vi "SIM control.vi"(11 "User":string="unknown-LAGSIM-user") -> ()   [LabVIEW 2018]
uses:
  <vilib>/DAQmx/write.llb/DAQmx Write (Digital Bool 1Line 1Point).vi
  <vilib>/DAQmx/create/channels.llb/DAQmx Create Channel (DO-Digital Output).vi
  <vilib>/DAQmx/write.llb/DAQmx Write (Analog DBL 1Chan 1Samp).vi
  <vilib>/DAQmx/write.llb/DAQmx Write (Digital 1D Bool 1Chan 1Samp).vi
  <vilib>/DAQmx/read.llb/DAQmx Read (Digital Bool 1Line 1Point).vi
  <vilib>/DAQmx/create/channels.llb/DAQmx Create Channel (AO-Voltage-Basic).vi
  <vilib>/DAQmx/read.llb/DAQmx Read (Analog DBL 1Chan 1Samp).vi
  <vilib>/Utility/file.llb/Write To Spreadsheet File (string).vi
  <vilib>/Utility/file.llb/Read From Spreadsheet File (string).vi
  <vilib>/Platform/browser.llb/Open URL in Default Browser (string).vi
  <vilib>/DAQmx/create/channels.llb/DAQmx Create Channel (AI-Voltage-Basic).vi
  <vilib>/Instr/_visa.llb/VISA Configure Serial Port (Instr).vi
  <vilib>/DAQmx/create/channels.llb/DAQmx Create Channel (DI-Digital Input).vi
panel:
  out "Laser Cluster":T1
  in  "y-move":bool
  in  "x-move":bool
  in  "y-rel (um)":dbl
  in  "x-rel (um)":dbl
  in  "Labstep API_Key":string="ZDNlNzY2YTYwNjk2YjY0Y2E4OGZhMGNiMDYxMWJkZjVjNWMwMjMzOQ=="
  in  "Live OS Channel Cluster":T2
  in  "Optosplit":bool
  in  "SIM Frames":i16=9
  in  "Bleach-\nsave ratio":dbl=1.0 min=0.0 max=1.0 step=0.1 format="%.2f"
  out "Current filter":string
  out "Current bookmark":i32
  out "TIRF Mode N":T3
  in  "Preview view":T4(radio)
  in  "Exposure\n(ms)":u32=100 min=1 max=2000 step=5
  in  "Channel":T5(radio)
  in  "Live on":bool
  out "Exposure times N":dbl[](array[numeric])
  out "Current piezo position (V)":dbl min=0.0 max=10.0 step=0.01 format="%_4g"
  out "ASI VISA resource name":refnum<visa-resource-name>="COM17"
  out "Voltage TIMEOUT (V)":dbl
  in  "stop":bool
  in  "Tab Control":T6(tab)=enum."-- Acquire --"
  in  "Clear table":bool
  in  "Create grid":bool
  in  "Load bkmk table":bool
  in  "Save bkmk table":bool
  in  "Delete bkmk":bool
  in  "Add bkmk":bool
  in  "Bookmark List":i32(listbox)=-1
  out "Output Voltage":dbl
  out "Total Sweep Images:":i16=360
  in  "Sweep Pattern":u8(ring)=21 items=["P9 0deg"=21, "P9 60deg"=22, "P9 120deg"=23, "P12 0deg"=24, "P12 60deg"=25, "P12 120deg"=26, "P15 0deg"=27, "P15 60deg"=28, "P15 120deg"=29]
  in  "Max V":dbl=1.0 min=-1.0 max=1.0
  in  "Min V":dbl=-1.0 min=-1.0 max=1.0
  in  "Sweep":bool caption="LCVR sweep"
  in  "V. steps":i16=40
  out "Step index:":i16
  in  "Voltages:":dbl[][](array[numeric])=[[0.09, 0.13, 0.16], [0.44, 0.52, 0.62], [-0.25, -0.28, -0.3]]
  in  "Filter Optosplit":i8=7 min=1 max=10 step=1
  in  "Filter 561":i8=3 min=1 max=10 step=1
  in  "Filter 640":i8=2 min=1 max=10 step=1
  in  "Filter 488":i8=4 min=1 max=10 step=1
  in  "Manual SLM mode":bool
  in  "RO":u8=7 max=41 step=1
  out "SLM status":i16
  out "RO #":u8=49
  out "SLM State":string="Active"
  in  "Z-move method":u16(ring)=1 items=["Analogue", "Serial"]
  out "Current RO":u8=7
  in  "use z offset":bool
  out "Current z-position (um)":dbl min=0.0 max=10.0 step=0.01 format="%_4g"
  in  "Z offset (um)":dbl[](array[numeric])=[0.0, -0.3, 84.0] min=0.0 max=360.0 step=0.1 format="%0.3f"
  out "Current z #":i16=1
  in  "z0 (um)":dbl step=0.01 format="%.2f"
  in  "Post to logbook":bool
  in  "Logbook entry":string
  in  "Open Logbook":bool
  in  "LED intensity":dbl min=0.0 max=100.0 step=1.0
  in  "ASI Unlock":bool
  in  "ASI Set Lock":bool
  in  "TIRF Info button":bool
  in  "640-OS":bool
  in  "561-OS":bool
  in  "488-OS":bool
  in  "Exp OS":string="100"
  in  "Ch3 TIRF":bool
  in  "Ch2 TIRF":bool
  in  "Ch1 TIRF":bool
  in  "Widefield?":bool
  in  "#bookmarks":i16 min=0 step=1
  in  "Acquire":bool
  in  "#Channels":i16=1 min=1 max=3 step=1
  in  "#t-frames":i16=1 min=1 step=1
  out "Total\nFrames":i16=36
  out "Current \nFrame":i32
  in  "Ch 1":T5(radio)
  in  "Ch 2":T5(radio)=enum."Radio Selection 2"
  in  "Ch 3":T5(radio)=enum."Radio Selection 3"
  in  "t-interval":u32 max=1000 step=1
  in  "Int unit":enum16{"ms", "s", "min"}(ring)
  in  "Exp 0":u32=100 caption="Exposure (ms) 2" min=1 max=2000 step=5
  in  "Exp 1":u32=100 caption="Exposure (ms) 2" min=1 max=2000 step=5
  in  "Exp 2":u32=100 caption="Exposure (ms) 2" min=1 max=2000 step=5
  in  "#z-planes":i16=1 min=1 step=1
  in  "z-step (um)":dbl=1.0
  out "Z move":bool
  out "Ch N":T7={"Ch 0"=enum."Radio Selection 1", "Ch 1"=enum."Radio Selection 2", "Ch 2"=enum."Radio Selection 3"}
  # "LIVE!"
  # "ADVANCED"
  # "Channel Variable Holders"
  # "Pockels Voltage Sweep"
  # "Pockels Voltage Settings"
  # "488           561            640"
  # "Rot 1\n\nRot 2\n\nRot 3"
  # "Filter position"
  # "ASI stage comms"
  # "488"
  # "640"
  # "Opto"
  # "561"
  # "Manual SLM control"
  # "Piezo offset"
  # "Channel #"
  # "Use this space to report any bugs, problems, or anything\nelse you like to the logbook."
  # "ASI Autofocus"
  # "UNDER DEVELOPMENT!!!"
  # "O/S"
  # "TIRF:"
  # "TIRF:"
  # "TIRF:"
  # "Wave-\nlength:"
  # "Exposure\ntime (ms):"
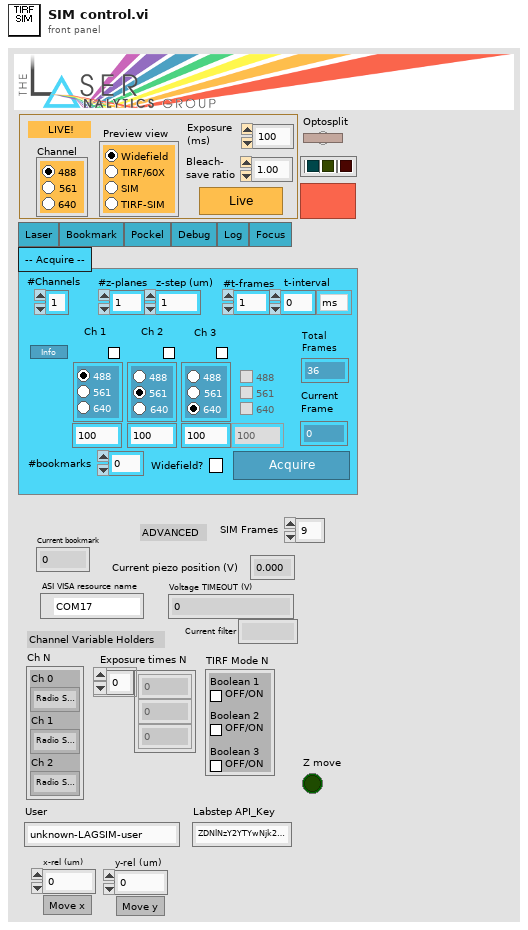
[diagram p1: front panel]
types:
  T1 = cluster{"488 indicator":bool, "488 indicator 3":bool, "488 indicator 2":bool}
  T2 = cluster{"488 OS live":bool, "640 OS live":bool, "561 OS live":bool}
  T3 = cluster{"Boolean 1":bool, "Boolean 2":bool, "Boolean 3":bool}
  T4 = enum32{"Radio Selection 1", "Radio Selection 2", "Radio Selection 3", "Radio Selection 4"}
  T5 = enum32{"Radio Selection 1", "Radio Selection 2", "Radio Selection 3"}
  T6 = enum32{"Laser", "Bookmark", "Pockel", "Debug", "Log", "Focus", "-- Acquire --"}
  T7 = cluster{"Ch 0":enum32{"Radio Selection 1", "Radio Selection 2", "Radio Selection 3"}, "Ch 1":enum32{"Radio Selection 1", "Radio Selection 2", "Radio Selection 3"}, "Ch 2":enum32{"Radio Selection 1", "Radio Selection 2", "Radio Selection 3"}}
  T8 = cluster{"Ch 1":enum32{"Radio Selection 1", "Radio Selection 2", "Radio Selection 3"}, "Ch 2":enum32{"Radio Selection 1", "Radio Selection 2", "Radio Selection 3"}, "Ch 3":enum32{"Radio Selection 1", "Radio Selection 2", "Radio Selection 3"}}
  T9 = cluster{"Ch1 TIRF":bool, "Ch2 TIRF":bool, "Ch3 TIRF":bool}
  T10 = cluster{"User":string, "Total\nFrames":i16, "#Channels":i16, "#t-frames":i16, "#z-planes":i16, "#bookmarks":i16, "Ch N":cluster{"Ch 0":enum32{"Radio Selection 1", "Radio Selection 2", "Radio Selection 3"}, "Ch 1":enum32{"Radio Selection 1", "Radio Selection 2", "Radio Selection 3"}, "Ch 2":enum32{"Radio Selection 1", "Radio Selection 2", "Radio Selection 3"}}, "Exposure times N":dbl[], "TIRF Mode N":cluster{"Boolean 1":bool, "Boolean 2":bool, "Boolean 3":bool}, "Optosplit":bool, "Widefield?":bool, "t-interval":u32, "RingText.Text":string, "z-step (um)":dbl, i32}
  T11 = enum8{"Enabled", "Disabled", "Disabled and Grayed Out"}
  T12 = cluster{"data[0]":bool, "data[1]":bool, "data[2]":bool}
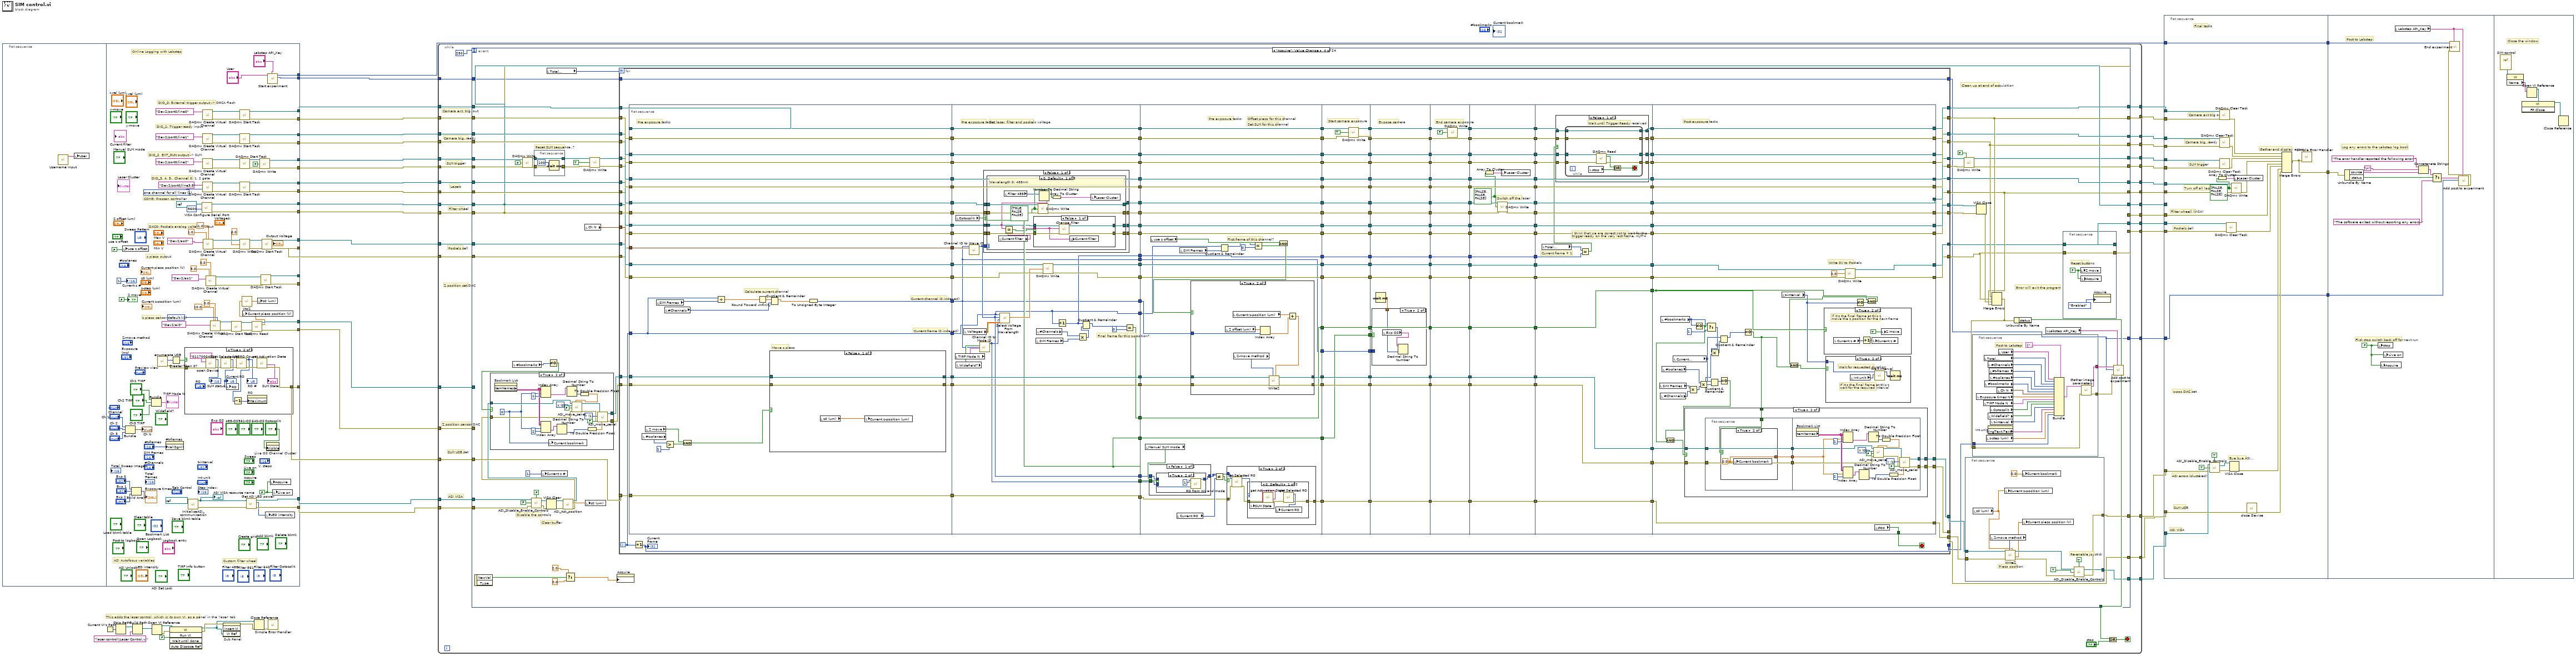
[diagram p0: block diagram]
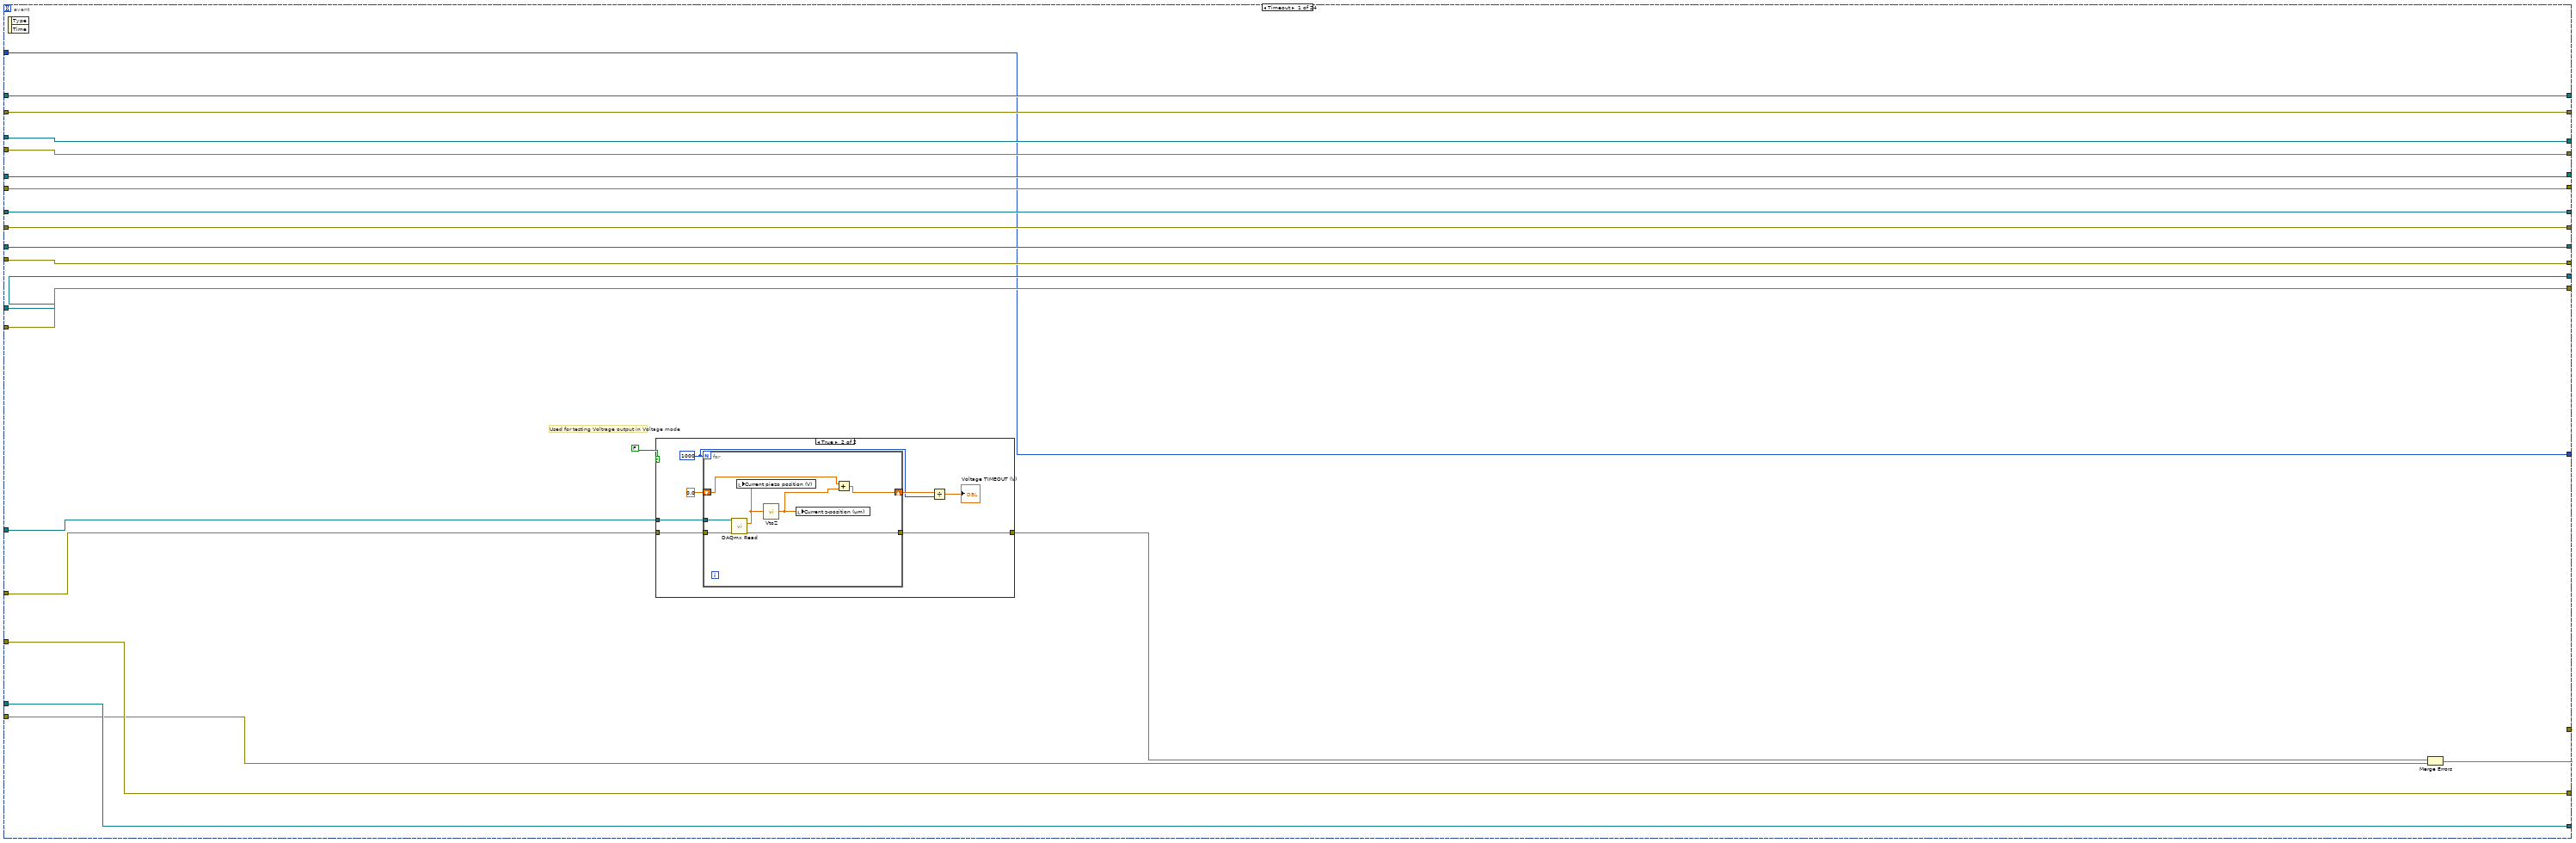
[diagram p2: hidden frame]
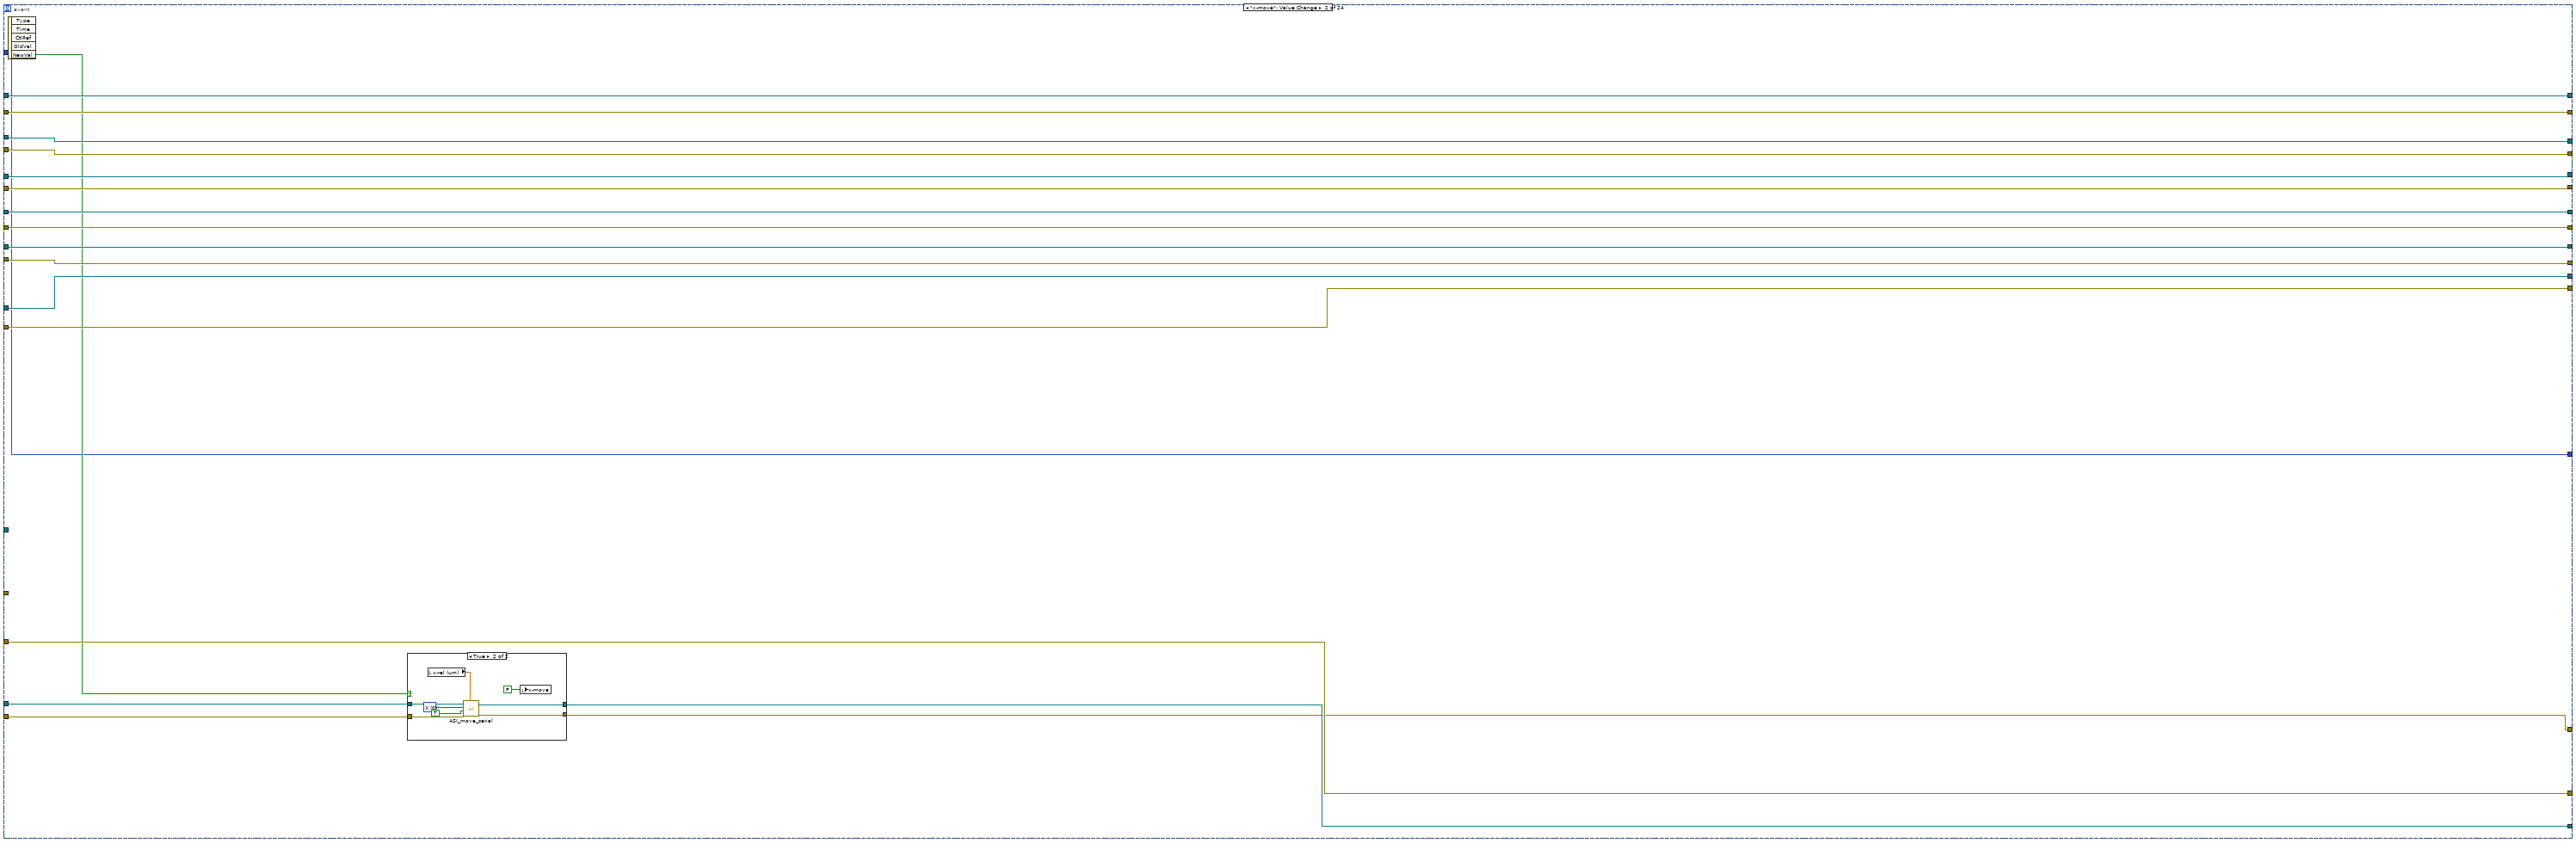
[diagram p4: hidden frame]
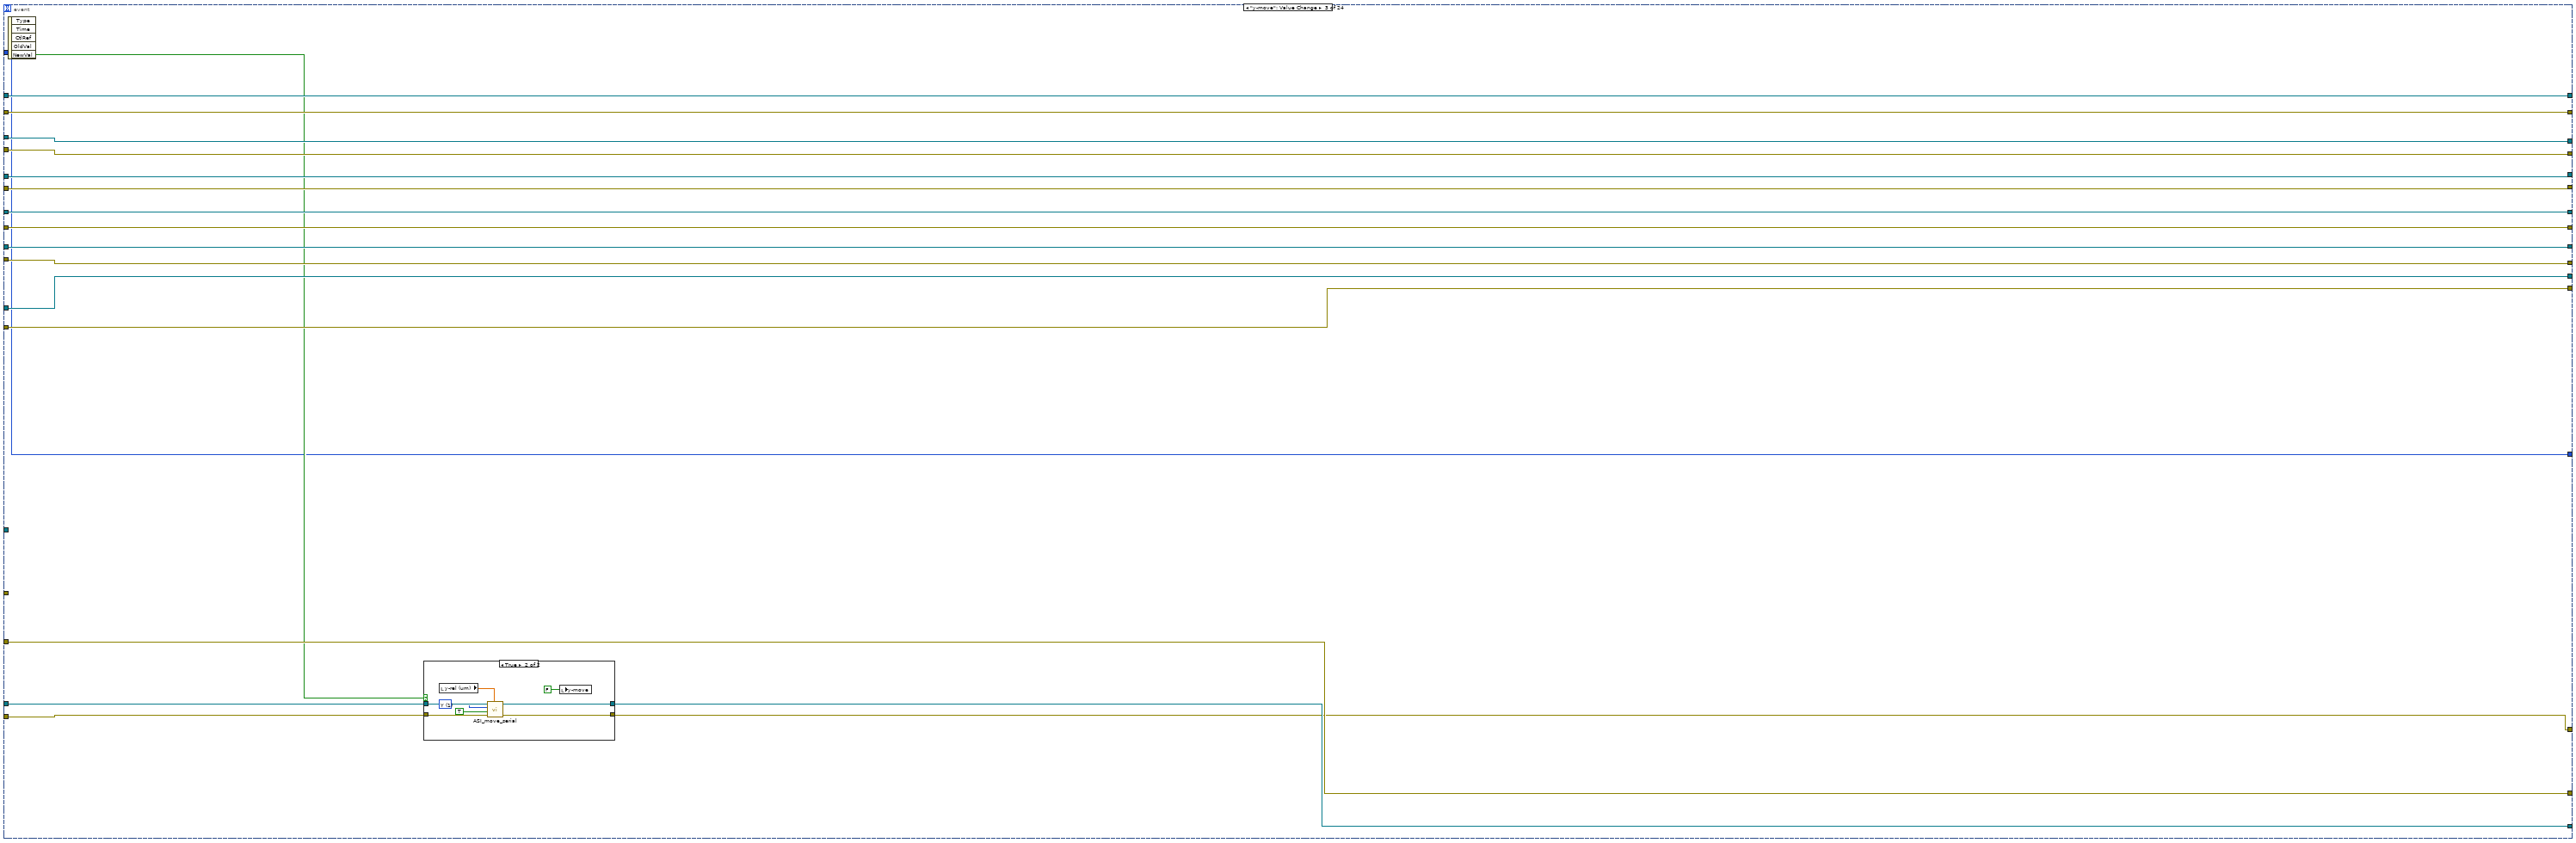
[diagram p6: hidden frame]
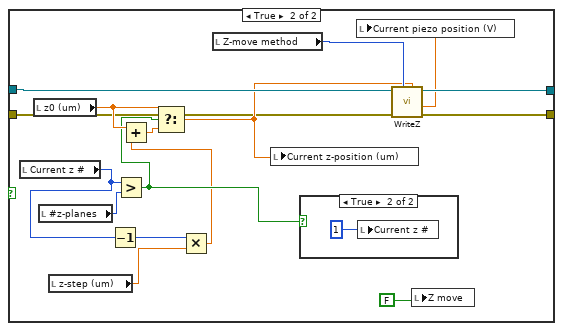
[diagram p9: hidden frame]
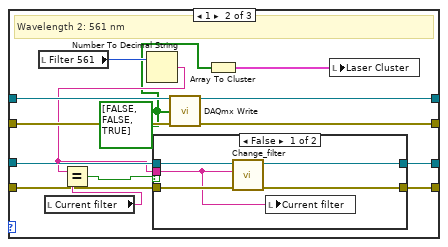
[diagram p12: hidden frame]
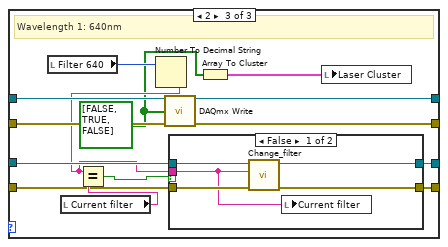
[diagram p14: hidden frame]
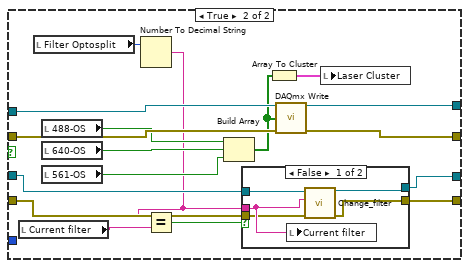
[diagram p16: hidden frame]
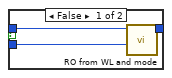
[diagram p20: hidden frame]
diagram:
  # "This adds the laser control, which is its own VI, as a panel in the 'laser' tab"
  n1 = flat-sequence {
    tunnel: [w136] -> w34
    tunnel: [w135] -> w48
    tunnel: [w131] -> w33
    tunnel: [w130] -> w46
    tunnel: [w121] -> w43
    tunnel: [w120] -> w42
    tunnel: [w111] -> w30
    tunnel: [w110] -> w39
    tunnel: [w109] -> w32
    tunnel: [w108] -> w36
    tunnel: [w99] -> w31
    tunnel: [w98] -> w35
    tunnel: [w81] -> w29
    tunnel: [w82] -> w28
    tunnel: [w88] -> _
    tunnel: [w87] -> _
    tunnel: [w75] -> w25
    tunnel: [w58] -> w24
    tunnel: [w56] -> w19
    tunnel: [w52] -> w1
    tunnel: [w51] -> w4
    frame #0 {
      n2 = call "Username Input.vi"() -> ("Username output"=w50:string)  [unwired: 11 in]
      n3 = local write "User"(w50) -> ()
    }
    frame #1 {
      w74 = FALSE ("Live mode")
      w91 = -1 items=["default"=-1, "RSE"=10083, "NRSE"=10078, "Differential"=10106, "Pseudodifferential"=12529] ("input terminal configuration")
      w106 = 1 items=["one channel for each line", "one channel for all lines"] ("line grouping")
      # "Custom filter wheel"
      # "ASI Autofocus variables"
      # "Online Logging with Labstep"
      # "z piezo sensor"
      # "z piezo output"
      # "COM5: Proscan controller"
      # "DIO_3, 4, 5:  Channel 0, 1, 2 gate"
      # "DIO_2  EXT_RUN output -> SLM"
      # "DAC0: Pockels analog voltage output"
      # "DIO_1: Trigger ready input"
      # "DIO_0: External trigger output -> ORCA Flash"
      n4 = local write "use z offset"(FALSE ("use z offset")) -> ()
      n5 = Bundle("Ch 1"="Ch 1", "Ch 2"="Ch 2", "Ch 3"="Ch 3") -> (→"Ch N":T8)  [unwired: 1 in]
      n6 = Build Array("Exp 0", "Exp 1", "Exp 2") -> (→"Exposure times N":u32[])
      n7 = Bundle("Ch1 TIRF"="Ch1 TIRF", "Ch2 TIRF"="Ch2 TIRF", "Ch3 TIRF"="Ch3 TIRF") -> (→"TIRF Mode N":T9)  [unwired: 1 in]
      n8 = call <userlib>:"enumerate USB.vi"() -> ("error out"=w76:errorcluster, "function return"=w78:i16)  [unwired: 9 in, 1 out]
      n9 = property on="#t-frames" class="DigNum (strict)"("Val(Sgnl)"="#t-frames") -> ()  [unwired: 2 in, 2 out]
      n10 = Greater Than 0?(x=w78) -> (x > 0?=w77:bool)
      n11 = case shown="True" w77 {
        tunnel: w76 -> [w141 w152]
        tunnel: [w140 w147] -> w75
        frame False {
          n12 = call <userlib>:"close Device.vi"("error in (no error)"=w141) -> ("error out"=w140:errorcluster)  [unwired: 9 in, 1 out]
        }
        frame True {
          n13 = call <userlib>:"open Device.vi"("error in (no error)"=w152, "identifier"="0117000451") -> ("error out"=w149:errorcluster, "function return"=→"SLM status":i16)  [unwired: 8 in]
          n14 = call <userlib>:"get Selected RO.vi"("error in (no error)"=w149) -> ("error out"=w148:errorcluster, "selectedRO"=w144:u8)  [unwired: 8 in, 1 out]
          "Current RO" <- w144
          n15 = local write "RO"(w144) -> ()
          n16 = call <userlib>:"get RO Count.vi"("error in (no error)"=w148) -> ("error out"=w146:errorcluster, "count"=w143:u8)  [unwired: 8 in, 1 out]
          "RO #" <- w143
          n17 = Decrement(x=w143) -> (x-1=w142:u8)
          n18 = property on="RO" class="DigNum (strict)"("Maximum"=w142) -> ()  [unwired: 2 in, 2 out]
          n19 = call <userlib>:"get Activation State.vi"("error in (no error)"=w146) -> ("error out"=w147:errorcluster, "String"=→"SLM State":string)  [unwired: 7 in, 2 out]
        }
      }
      n20 = call "InitialiseASI_communication.vi"("COM port"=refnum<visa-resource-name> "COM17") -> ("error out"=w57:errorcluster, "VISA resource name out"=w59:refnum<visa-resource-name>)  [unwired: 3 in]
      "ASI VISA resource name" <- w59
      n21 = call-poly "VISA Configure Serial Port"("VISA resource name"=refnum<visa-resource-name> "COM5", "baud rate (9600)"=u32 9600) -> ("VISA resource name out"=w99:refnum<visa-resource-name>, "error out"=w98:errorcluster)  [unwired: 12 in]
      n22 = call-poly <vilib>:"DAQmx Create Virtual Channel.vi"("lines"=tag "Dev2/port0/line0") -> ("task out"=w138:refnum<k21>, "error out"=w139:errorcluster)  [unwired: 13 in]
      n23 = call-poly <vilib>:"DAQmx Create Virtual Channel.vi"("lines"=tag "Dev2/port0/line1") -> ("task out"=w133:refnum<k21>, "error out"=w132:errorcluster)  [unwired: 13 in]
      n24 = call-poly <vilib>:"DAQmx Create Virtual Channel.vi"("lines"=tag "Dev2/port0/line2") -> ("task out"=w118:refnum<k21>, "error out"=w117:errorcluster)  [unwired: 13 in]
      n25 = call-poly <vilib>:"DAQmx Create Virtual Channel.vi"("lines"="Dev2/port0/line3:5", "line grouping"=w106) -> ("task out"=w116:refnum<k21>, "error out"=w115:errorcluster)  [unwired: 12 in]
      n26 = call-poly <vilib>:"DAQmx Create Virtual Channel.vi"("maximum value"=1.0, "minimum value"=-1.0, "physical channels"=tag "Dev2/ao0") -> ("task out"=w124:refnum<k21>, "error out"=w123:errorcluster)  [unwired: 11 in]
      n27 = call-poly <vilib>:"DAQmx Create Virtual Channel.vi"("maximum value"=5.0, "minimum value"=0.0, "physical channels"=tag "Dev2/ao1") -> ("task out"=w94:refnum<k21>, "error out"=w93:errorcluster)  [unwired: 11 in]
      n28 = call-poly <vilib>:"DAQmx Create Virtual Channel.vi"("maximum value"=10.0, "minimum value"=0.0, "input terminal configuration"=w91, "physical channels"=tag "Dev2/ai0" ("Physical Channel")) -> ("task out"=w86:refnum<k21>, "error out"=w85:errorcluster)  [unwired: 10 in]
      n29 = call <vilib>:"DAQmx Start Task.vi"("task/channels in"=w86, "error in"=w85) -> ("task out"=w84:refnum<k21>, "error out"=w83:errorcluster)  [unwired: 12 in]
      n30 = call <vilib>:"DAQmx Start Task.vi"("task/channels in"=w138, "error in"=w139) -> ("task out"=w136:refnum<k21>, "error out"=w135:errorcluster)  [unwired: 12 in]
      n31 = call <vilib>:"DAQmx Start Task.vi"("task/channels in"=w133, "error in"=w132) -> ("task out"=w131:refnum<k21>, "error out"=w130:errorcluster)  [unwired: 12 in]
      n32 = call <vilib>:"DAQmx Start Task.vi"("task/channels in"=w118, "error in"=w117) -> ("task out"=w114:refnum<k21>, "error out"=w113:errorcluster)  [unwired: 12 in]
      n33 = call <vilib>:"DAQmx Start Task.vi"("task/channels in"=w116, "error in"=w115) -> ("task out"=w109:refnum<k21>, "error out"=w108:errorcluster)  [unwired: 12 in]
      n34 = call-poly <vilib>:"DAQmx Write.vi"("task/channels in"=w124, "data"=0.0, "error in"=w123) -> ("task out"=w128:refnum<k21>, "error out"=w127:errorcluster)  [unwired: 10 in, 1 out]
      n35 = call "Get ASI LED power.vi"("error in"=w57, "VISA resource in"=w59) -> ("error out"=w56:errorcluster, "LED power"=w55:i32, "VISA resource name out"=w58:refnum<visa-resource-name>)  [unwired: 7 in]
      n36 = call-poly <vilib>:"DAQmx Read.vi"("task/channels in"=w84, "error in"=w83) -> ("task out"=w81:refnum<k21>, "data"=w79:dbl, "error out"=w82:errorcluster)  [unwired: 11 in]
      n37 = call "VtoZ.vi"("Voltage IN"=w79) -> ("Zpos OUT (um)"=w72:dbl)
      n38 = local write "Current piezo position (V)"(w79) -> ()
      n39 = local write "z0 (um)"(w72) -> ()
      n40 = call-poly <vilib>:"DAQmx Write.vi"("task/channels in"=w114, "data"=FALSE, "error in"=w113) -> ("task out"=w111:refnum<k21>, "error out"=w110:errorcluster)  [unwired: 10 in, 1 out]
      n41 = call <vilib>:"DAQmx Start Task.vi"("task/channels in"=w94, "error in"=w93) -> ("task out"=w88:refnum<k21>, "error out"=w87:errorcluster)  [unwired: 12 in]
      n42 = call <vilib>:"DAQmx Start Task.vi"("task/channels in"=w128, "error in"=w127) -> ("task out"=w121:refnum<k21>, "error out"=w120:errorcluster)  [unwired: 12 in]
      n43 = local write "LED intensity"(w55) -> ()
      n44 = property on="Live OS Channel Cluster" class="Clust (strict)"("Visible"="Optosplit") -> ()  [unwired: 2 in, 2 out]
      n45 = call "Start experiment.vi"("API Key"="Labstep API_Key", "Name of LAG SIM user"="User") -> ("Thread ID"=w51:i32, "Experiment ID"=w52:i32)  [unwired: 7 in, 1 out]
      n46 = local write "Acquire"(w74) -> ()
      n47 = local write "Live on"(w74) -> ()
      "Current z #" <- i16 1 ("Current z #")
      "Z move" <- FALSE ("Z move")
    }
  }
  n48 = Current VI's Path() -> (path=w14:path)
  n49 = Strip Path(path=w14) -> (stripped path=w12:path)  [unwired: 1 out]
  n50 = Build Path(base path=w12, name or relative path="laser control\\Laser Control.vi") -> (appended path=w13:path)
  n51 = Open VI Reference(vi path=w13) -> (vi reference=w17:refnum<vi>, error out=w16:errorcluster)  [unwired: 5 in]
  n52 = invoke class="VI" method="Run VI"(reference=w17, error in=w16, "Wait until done"=FALSE) -> (reference out=w7:refnum<vi>, error out=w9:errorcluster)  [unwired: 2 in, 3 out]
  n53 = invoke on="Sub Panel" class="SubPanel" method="Insert VI"(error in=w9, "VI Ref"=w7) -> (error out=w8:errorcluster)  [unwired: 2 in, 3 out]
  n54 = Close Reference(reference=w7, error in (no error)=w8) -> (error out=w11:errorcluster)
  n55 = call <vilib>:"Simple Error Handler.vi"("error in (no error)"=w11) -> ()  [unwired: 4 in, 5 out]
  n56 = while {
    tunnel: w34 -> [w190]
    tunnel: [w189] -> w49
    tunnel: w48 -> [w188]
    tunnel: [w187] -> w47
    tunnel: w33 -> [w186]
    tunnel: w46 -> [w185]
    tunnel: [w184] -> w45
    tunnel: [w168] -> w44
    tunnel: w43 -> [w183]
    tunnel: w42 -> [w182]
    tunnel: [w181] -> w41
    tunnel: [w180] -> w40
    tunnel: w30 -> [w179]
    tunnel: w39 -> [w178]
    tunnel: [w177] -> w37
    tunnel: [w176] -> w38
    tunnel: w32 -> [w175]
    tunnel: w36 -> [w174]
    tunnel: w31 -> [w173]
    tunnel: w35 -> [w172]
    tunnel: w29 -> [w171]
    tunnel: w28 -> [w170]
    tunnel: [w169] -> w27
    tunnel: [w166] -> w26
    tunnel: w25 -> [w167]
    tunnel: w24 -> [w164]
    tunnel: [w163] -> w23
    tunnel: [w162] -> w22
    tunnel: [w158] -> w21
    tunnel: [w157] -> w20
    tunnel: w19 -> [w156]
    tunnel: [w155] -> w18
    tunnel: w4 -> [w154]
    tunnel: [w153] -> w3
    stop <- w161 stop-if-true
    # "Camera trig. ready"
    # "Camera ext. trig. out"
    # "SLM trigger"
    # "Lasers"
    # "SLM USB set"
    # "Filter wheel"
    # "Pockels cell"
    # "ASI VISA"
    # "Z position sensor DAC"
    # "Z position set DAC"
    n57 = event shown="[3] \"Acquire\": Value Change" {
      selector: _ -> [_ _ _ _ _ _ _ _ _ _ _ _ _ _ _ _ _ _ _ _ _ _ _ _]
      dyn-events: _ -> [_ _ _ _ _ _ _ _ _ _ _ _ _ _ _ _ _ _ _ _ _ _ _ _]
      timeout: 250 -> [_ _ _ _ _ _ _ _ _ _ _ _ _ _ _ _ _ _ _ _ _ _ _ _]
      tunnel: w190 -> [w195 w245 w274 w358 w1092 w1130 w1528 w1578 w2099 w2102 w2128 w2162 w2190 w2230 w2285 w2305 w2322 w2352 w2370 w2394 w2423 w2449 w2474 w2492]
      tunnel: [w195 w245 w274 w356 w1092 w1114 w1528 w1574 w2099 w2102 w2128 w2162 w2190 w2230 w2285 w2305 w2322 w2352 w2370 w2394 w2423 w2449 w2474 w2492] -> w189
      tunnel: w188 -> [w196 w244 w273 w357 w1091 w1129 w1529 w1577 w2098 w2103 w2129 w2163 w2191 w2229 w2284 w2304 w2321 w2351 w2369 w2393 w2422 w2448 w2473 w2491]
      tunnel: [w196 w244 w273 w353 w1091 w1101 w1529 w1573 w2098 w2103 w2129 w2163 w2191 w2229 w2284 w2304 w2321 w2351 w2369 w2393 w2422 w2448 w2473 w2491] -> w187
      tunnel: w186 -> [w197 w242 w271 w355 w1089 w1128 w1530 w1576 w2096 w2104 w2130 w2164 w2192 w2227 w2282 w2302 w2319 w2349 w2367 w2391 w2420 w2446 w2471 w2489]
      tunnel: w185 -> [w198 w243 w272 w354 w1090 w1127 w1531 w1575 w2097 w2105 w2131 w2165 w2193 w2228 w2283 w2303 w2320 w2350 w2368 w2392 w2421 w2447 w2472 w2490]
      tunnel: [w198 w243 w272 w352 w1090 w1096 w1531 w1571 w2097 w2105 w2131 w2165 w2193 w2228 w2283 w2303 w2320 w2350 w2368 w2392 w2421 w2447 w2472 w2490] -> w184
      tunnel: [w197 w242 w271 w351 w1089 w1098 w1530 w1572 w2096 w2104 w2130 w2164 w2192 w2227 w2282 w2302 w2319 w2349 w2367 w2391 w2420 w2446 w2471 w2489] -> w168
      tunnel: w183 -> [w203 w241 w270 w349 w1088 w1136 w1538 w1559 w2095 w2112 w2138 w2172 w2200 w2226 w2281 w2301 w2318 w2348 w2366 w2390 w2419 w2445 w2470 w2488]
      tunnel: w182 -> [w204 w240 w269 w348 w1087 w1135 w1539 w1557 w2094 w2113 w2139 w2173 w2201 w2225 w2280 w2300 w2317 w2347 w2365 w2389 w2418 w2444 w2469 w2487]
      tunnel: [w203 w241 w270 w314 w1088 w1121 w1538 w1558 w2095 w2112 w2138 w2172 w2200 w2226 w2281 w2301 w2318 w2348 w2366 w2390 w2419 w2445 w2470 w2488] -> w181
      tunnel: [w204 w240 w269 w315 w1087 w1120 w1539 w1556 w2094 w2113 w2139 w2173 w2201 w2225 w2280 w2300 w2317 w2347 w2365 w2389 w2418 w2444 w2469 w2487] -> w180
      tunnel: w179 -> [w199 w238 w267 w332 w1085 w1138 w1532 w1580 w2092 w2106 w2132 w2166 w2194 w2223 w2278 w2298 w2315 w2345 w2363 w2387 w2416 w2442 w2467 w2485]
      tunnel: w178 -> [w200 w239 w268 w331 w1086 w1137 w1533 w1579 w2093 w2107 w2133 w2167 w2195 w2224 w2279 w2299 w2316 w2346 w2364 w2388 w2417 w2443 w2468 w2486]
      tunnel: [w200 w239 w268 w334 w1086 w1097 w1533 w1569 w2093 w2107 w2133 w2167 w2195 w2224 w2279 w2299 w2316 w2346 w2364 w2388 w2417 w2443 w2468 w2486] -> w177
      tunnel: [w199 w238 w267 w336 w1085 w1100 w1532 w1570 w2092 w2106 w2132 w2166 w2194 w2223 w2278 w2298 w2315 w2345 w2363 w2387 w2416 w2442 w2467 w2485] -> w176
      tunnel: w175 -> [w207 w236 w265 w344 w1082 w1134 w1534 w1584 w2090 w2108 w2134 w2168 w2196 w2221 w2275 w2295 w2312 w2342 w2360 w2384 w2414 w2440 w2465 w2482]
      tunnel: w174 -> [w206 w235 w264 w343 w1081 w1133 w1535 w1581 w2089 w2109 w2135 w2169 w2197 w2220 w2274 w2294 w2311 w2341 w2359 w2383 w2413 w2439 w2464 w2481]
      tunnel: w173 -> [w201 w233 w262 w341 w1079 w1132 w1536 w1583 w2087 w2110 w2136 w2170 w2198 w2218 w2272 w2292 w2309 w2339 w2357 w2381 w2411 w2437 w2462 w2479]
      tunnel: w172 -> [w202 w234 w263 w340 w1080 w1131 w1537 w1582 w2088 w2111 w2137 w2171 w2199 w2219 w2273 w2293 w2310 w2340 w2358 w2382 w2412 w2438 w2463 w2480]
      tunnel: w171 -> [w210 _ _ _ _ _ _ _ _ _ _ _ _ _ _ _ _ _ _ _ _ _ _ _]
      tunnel: w170 -> [w209 _ _ _ _ _ _ _ _ _ _ _ _ _ _ _ _ _ _ _ _ _ _ _]
      tunnel: [w192 w231 w258 w320 w1084 w1104 w1540 w1552 w2081 w2114 w2140 w2174 w2202 w2210 w2277 w2297 w2314 w2344 w2362 w2386 w2407 w2433 w2458 w2484] -> w169
      tunnel: w167 -> [w211 w237 w266 w305 w1083 w1107 w1541 w1560 w2091 w2119 w2141 w2175 w2204 w2222 w2276 w2296 w2313 w2343 w2361 w2385 w2415 w2441 w2466 w2483]
      tunnel: [w211 w237 w266 w304 w1083 w1106 w1541 w1561 w2091 w2120 w2141 w2175 w2204 w2222 w2276 w2296 w2313 w2343 w2361 w2385 w2415 w2441 w2466 w2483] -> w166
      tunnel: w164 -> [w205 w229 w261 w323 w1078 w1105 w1542 w1555 w2080 w2115 w2142 w2176 w2208 w2213 w2271 w2291 w2308 w2338 w2356 w2380 w2406 w2432 w2461 w2478]
      tunnel: [w207 w236 w265 w318 w1082 w1112 w1534 w1568 w2090 w2108 w2134 w2168 w2196 w2221 w2275 w2295 w2312 w2342 w2360 w2384 w2414 w2440 w2465 w2482] -> w163
      tunnel: [w206 w235 w264 w317 w1081 w1113 w1535 w1567 w2089 w2109 w2135 w2169 w2197 w2220 w2274 w2294 w2311 w2341 w2359 w2383 w2413 w2439 w2464 w2481] -> w162
      tunnel: [_ _ _ w316 _ _ _ _ _ _ _ _ _ _ _ _ _ _ _ _ _ _ _ _] -> w159
      tunnel: [w202 w234 w263 w340 w1080 w1110 w1537 w1566 w2088 w2111 w2137 w2171 w2199 w2219 w2273 w2293 w2310 w2340 w2358 w2382 w2412 w2438 w2463 w2480] -> w158
      tunnel: [w201 w233 w262 w341 w1079 w1109 w1536 w1565 w2087 w2110 w2136 w2170 w2198 w2218 w2272 w2292 w2309 w2339 w2357 w2381 w2411 w2437 w2462 w2479] -> w157
      tunnel: w156 -> [w194 w230 w259 w303 w1084 w1104 w1540 w1554 w2082 w2114 w2140 w2174 w2189 w2211 w2277 w2297 w2314 w2344 w2362 w2386 w2408 w2434 w2459 w2484]
      tunnel: [w205 w232 w260 w301 w1078 w1105 w1542 w1553 w2079 w2115 w2142 w2176 w2203 w2212 w2271 w2291 w2308 w2338 w2356 w2380 w2405 w2431 w2460 w2478] -> w155
      tunnel: w154 -> [w191 w227 w256 w290 w1071 w1093 w1527 w1550 w2073 w2101 w2127 w2155 w2188 w2209 w2268 w2286 w2307 w2332 w2353 w2372 w2404 w2430 w2456 w2475]
      tunnel: [w191 w227 w256 w285 w1071 w1093 w1527 w1550 w2073 w2101 w2127 w2155 w2188 w2209 w2268 w2286 w2307 w2332 w2353 w2372 w2404 w2430 w2456 w2475] -> w153
      event Timeout {
        # "Used for testing Voltrage output in Voltage mode"
        n58 = event-data() -> ()  [unwired: 1 in, 2 out]
        n59 = case shown="True" FALSE ("Auto Z") {
          tunnel: w210 -> [_ w219]
          tunnel: w209 -> [w212 w218]
          tunnel: [w212 w213] -> w193
          frame False {
          }
          frame True {
            w216 = 1000
            n60 = for {
              N: w216 -> [_]
              tunnel: w219 -> [w225]
              tunnel: w218 -> [w224]
              shift-right: [w222] -> w217
              shift-left: 0.0 -> [w221]
              tunnel: [w220] -> w213
              n61 = call-poly <vilib>:"DAQmx Read.vi"("task/channels in"=w225, "error in"=w224) -> ("data"=w226:dbl, "error out"=w220:errorcluster)  [unwired: 11 in, 1 out]
              n62 = local write "Current piezo position (V)"(w226) -> ()
              n63 = call "VtoZ.vi"("Voltage IN"=w226) -> ("Zpos OUT (um)"=w223:dbl)
              n64 = local write "Current z-position (um)"(w223) -> ()
              n65 = Add(x=w221, y=w223) -> (x+y=w222:dbl)
            }
            n66 = Divide(x=w217, y=w216) -> (x/y=→"Voltage TIMEOUT (V)":dbl)
          }
        }
        n67 = Merge Errors(w193, w194) -> (w192:errorcluster)
      }
      event "x-move": Value Change {
        n68 = event-data() -> ("NewVal"=w228:bool)  [unwired: 1 in, 4 out]
        n69 = case shown="True" w228 {
          tunnel: [w247 w255] -> w232
          tunnel: [w246 w254] -> w231
          tunnel: w230 -> [w246 w253]
          tunnel: w229 -> [w247 w251]
          frame False {
          }
          frame True {
            w250 = u16 0 items=["X", "Y", "Z"] ("Axis")
            n70 = local read "x-rel (um)"() -> (w249:dbl)
            n71 = call "ASI_move_serial.vi"("Position/distance (um)"=w249, "error in"=w253, "Relative?"=TRUE, "Axis"=w250, "VISA resource name"=w251) -> ("error out"=w254:errorcluster, "VISA resource name out"=w255:refnum<visa-resource-name>)  [unwired: 2 in]
            n72 = local write "x-move"(FALSE ("x-move")) -> ()
          }
        }
      }
      event "y-move": Value Change {
        n73 = event-data() -> ("NewVal"=w257:bool)  [unwired: 1 in, 4 out]
        n74 = case shown="True" w257 {
          tunnel: w261 -> [w276 w284]
          tunnel: [w276 w283] -> w260
          tunnel: w259 -> [w275 w282]
          tunnel: [w275 w281] -> w258
          frame False {
          }
          frame True {
            w280 = u16 1 items=["X", "Y", "Z"] ("Axis")
            n75 = local read "y-rel (um)"() -> (w278:dbl)
            n76 = call "ASI_move_serial.vi"("Position/distance (um)"=w278, "error in"=w282, "Relative?"=TRUE, "Axis"=w280, "VISA resource name"=w284) -> ("error out"=w281:errorcluster, "VISA resource name out"=w283:refnum<visa-resource-name>)  [unwired: 2 in]
            n77 = local write "y-move"(FALSE ("y-move")) -> ()
          }
        }
      }
      event "Acquire": Value Change {
        # "Error will exit the program"
        # "Reset SLM sequence..?"
        # "Clean up at end of acquisition"
        # "Clear buffer"
        # "Disable the controls"
        n78 = event-data() -> ("NewVal"=w312:bool)  [unwired: 1 in, 1 out]
        n79 = local read "#bookmarks"() -> (w297:i16)
        n80 = call-poly <vilib>:"DAQmx Write.vi"("task/channels in"=w332, "data"=FALSE, "error in"=w331) -> ("task out"=w327:refnum<k21>, "error out"=w329:errorcluster)  [unwired: 10 in, 1 out]
        n81 = call "ASI_Disable_Enable_Controls.vi"("Enable Z"=FALSE ("Disable Z"), "error in"=w303, "Enable XY"=FALSE ("Disable XY"), "VISA resource name"=w323) -> ("error out"=w302:errorcluster, "VISA resource name out"=w319:refnum<visa-resource-name>)
        n82 = flat-sequence {
          tunnel: [w419] -> w330
          tunnel: w329 -> [w419]
          tunnel: [w418] -> w328
          tunnel: w327 -> [w418]
          frame #0 {
            n83 = Wait (ms)(milliseconds to wait=u32 100) -> ()  [unwired: 1 out]
          }
        }
        n84 = local write "Current z #"(i16 1 ("z #")) -> ()
        n85 = VISA Clear(VISA resource name=w319, error in (no error)=w302) -> (VISA resource name out=w300:refnum<visa-resource-name>, error out=w299:errorcluster)
        n86 = local read "Total\nFrames"() -> (w350:i16)
        n87 = Not Equal To 0?(x=w297) -> (x != 0?=w296:bool)
        n88 = call "ASI_Ask_position.vi"("error in"=w299, "VISA resource name"=w300) -> ("error out"=w292:errorcluster, "Current Z position (um)"=w298:dbl, "VISA resource name out"=w295:refnum<visa-resource-name>)  [unwired: 7 in]
        n89 = case shown="True" w296 {
          tunnel: w295 -> [w379 w385]
          tunnel: [w379 w384] -> w294
          tunnel: [w380 w383] -> w293
          tunnel: w292 -> [w380 w382]
          frame False {
          }
          frame True {
            w381 = 0 ("index (row)")
            w393 = u16 1 items=["X", "Y", "Z"] ("Axis")
            w400 = u16 0 items=["X", "Y", "Z"] ("Axis")
            n90 = property on="Bookmark List" class="MCListbox (strict)"() -> ("ItemNames"=w397:string[][])  [unwired: 2 in, 2 out]
            n91 = Index Array(array=w397, index (row)=w381, index (col)=1 ("disabled index (col)")) -> (element=w396:string)
            n92 = Index Array(array=w397, index (row)=w381, index (col)=2 ("disabled index (col)")) -> (element=w391:string)
            n93 = local write "Current bookmark"(w381) -> ()
            n94 = Decimal String To Number(string=w391) -> (number=w386:i32)  [unwired: 2 in, 1 out]
            n95 = Decimal String To Number(string=w396) -> (number=w389:i32)  [unwired: 2 in, 1 out]
            n96 = To Double Precision Float(number=w389) -> (double precision float=w388:dbl)
            n97 = call "ASI_move_serial.vi"("Position/distance (um)"=w388, "error in"=w382, "Relative?"=FALSE, "Axis"=w400, "VISA resource name"=w385) -> ("error out"=w390:errorcluster, "VISA resource name out"=w394:refnum<visa-resource-name>)  [unwired: 2 in]
            n98 = To Double Precision Float(number=w386) -> (double precision float=w387:dbl)
            n99 = call "ASI_move_serial.vi"("Position/distance (um)"=w387, "error in"=w390, "Relative?"=FALSE, "Axis"=w393, "VISA resource name"=w394) -> ("error out"=w383:errorcluster, "VISA resource name out"=w384:refnum<visa-resource-name>)  [unwired: 2 in]
          }
        }
        n100 = Select(t=2.0, s=w312, f=0.0) -> (s? t:f=w311:dbl)
        n101 = local read "Ch N"() -> (w342:T7)
        n102 = local write "z0 (um)"(w298) -> ()
        n103 = call-poly <vilib>:"DAQmx Write.vi"("task/channels in"=w328, "data"=TRUE, "error in"=w330) -> ("task out"=w346:refnum<k21>, "error out"=w345:errorcluster)  [unwired: 10 in, 1 out]
        n104 = property on="Acquire" class="Bool (strict)"("DisabledEnum"=w311) -> ()  [unwired: 2 in, 2 out]
        n105 = for {
          N: w350 -> [_]
          tunnel: w358 -> [w601]
          tunnel: w357 -> [w600]
          tunnel: [w599] -> w356
          tunnel: [w598] -> w353
          tunnel: w355 -> [w597]
          tunnel: w354 -> [w596]
          tunnel: [w595] -> w352
          tunnel: [w594] -> w351
          tunnel: w349 -> [w592]
          tunnel: w348 -> [w591]
          tunnel: [w590] -> w306
          tunnel: [w589] -> w307
          tunnel: [w582] -> w337
          tunnel: w346 -> [w580]
          tunnel: [w579] -> w335
          tunnel: w345 -> [w577]
          tunnel: w344 -> [w576]
          tunnel: w343 -> [w575]
          tunnel: w342 -> [w574]
          tunnel: w341 -> [w548]
          tunnel: w340 -> [w547]
          tunnel: [w546] -> w339
          tunnel: [w501] -> w325
          tunnel: w294 -> [w497]
          tunnel: [w491] -> w324
          tunnel: [w489] -> w318
          tunnel: [w488] -> w317
          tunnel: [w479] -> w309
          tunnel: w305 -> [w469]
          tunnel: [w463] -> w304
          tunnel: w293 -> [w462]
          tunnel: w290 -> [w421]
          tunnel: [w421] -> w285
          tunnel: [w420] -> w286
          i -> [w593]
          stop <- w484 stop-if-true
          n106 = flat-sequence {
            tunnel: w547 -> [w619]
            tunnel: w548 -> [w620]
            tunnel: w574 -> [w621]
            tunnel: w575 -> [w622]
            tunnel: w576 -> [w623]
            tunnel: w577 -> [w624]
            tunnel: w580 -> [w625]
            tunnel: w591 -> [w626]
            tunnel: w592 -> [w627]
            tunnel: w593 -> [w609]
            tunnel: w596 -> [w628]
            tunnel: w597 -> [w629]
            tunnel: w600 -> [w630]
            tunnel: w601 -> [w631]
            tunnel: [w631] -> w518
            tunnel: [w630] -> w517
            tunnel: [w629] -> w516
            tunnel: [w628] -> w515
            tunnel: [w609] -> w514
            tunnel: [w627] -> w513
            tunnel: [w626] -> w512
            tunnel: [w625] -> w511
            tunnel: [w624] -> w510
            tunnel: [w623] -> w509
            tunnel: [w622] -> w508
            tunnel: [w621] -> w507
            tunnel: [w620] -> w506
            tunnel: [w619] -> w505
            tunnel: [w613] -> w502
            tunnel: w497 -> [w612]
            tunnel: [w611] -> w495
            tunnel: [w606] -> w487
            tunnel: [w603] -> w470
            tunnel: w469 -> [w603]
            tunnel: w462 -> [w602]
            tunnel: [w689] -> w542
            tunnel: [w688] -> w540
            tunnel: [w687] -> w538
            tunnel: [w686] -> w536
            tunnel: [w672] -> w534
            tunnel: [w670] -> w532
            tunnel: [w685] -> w530
            tunnel: [w684] -> w528
            tunnel: [w667] -> w526
            tunnel: [w680] -> w524
            tunnel: [w679] -> w522
            tunnel: [w676] -> w520
            tunnel: w518 -> [w689]
            tunnel: w517 -> [w688]
            tunnel: w516 -> [w687]
            tunnel: w515 -> [w686]
            tunnel: w514 -> [w652]
            tunnel: w513 -> [w673]
            tunnel: w512 -> [w671]
            tunnel: w511 -> [w685]
            tunnel: w510 -> [w684]
            tunnel: w509 -> [w683]
            tunnel: w508 -> [w682]
            tunnel: w507 -> [w681]
            tunnel: w506 -> [w678]
            tunnel: w505 -> [w677]
            tunnel: [w675] -> w503
            tunnel: w502 -> [w675]
            tunnel: [w674] -> w496
            tunnel: w495 -> [w674]
            tunnel: w487 -> [w653]
            tunnel: [w661] -> w480
            tunnel: [w660] -> w474
            tunnel: [w653] -> w473
            tunnel: [w659] -> w472
            tunnel: [w656] -> w471
            tunnel: w470 -> [w658]
            tunnel: [w658] -> w468
            tunnel: [w654] -> w427
            tunnel: [w654] -> w426
            tunnel: [w653] -> w423
            tunnel: [w652] -> w422
            tunnel: w542 -> [w819]
            tunnel: [w819] -> w541
            tunnel: w540 -> [w818]
            tunnel: [w818] -> w539
            tunnel: w538 -> [w817]
            tunnel: [w817] -> w537
            tunnel: w536 -> [w816]
            tunnel: [w816] -> w535
            tunnel: w534 -> [w815]
            tunnel: [w815] -> w533
            tunnel: w532 -> [w814]
            tunnel: [w814] -> w531
            tunnel: w530 -> [w813]
            tunnel: [w813] -> w529
            tunnel: w528 -> [w812]
            tunnel: [w812] -> w527
            tunnel: w526 -> [w802]
            tunnel: [w802] -> w525
            tunnel: w524 -> [w811]
            tunnel: [w811] -> w523
            tunnel: w522 -> [w810]
            tunnel: [w810] -> w521
            tunnel: w520 -> [w809]
            tunnel: [w809] -> w519
            tunnel: w503 -> [w807]
            tunnel: [w806] -> w498
            tunnel: w496 -> [w804]
            tunnel: [w803] -> w492
            tunnel: [w801] -> w485
            tunnel: [w800] -> w481
            tunnel: w480 -> [w800]
            tunnel: [w799] -> w475
            tunnel: w474 -> [w799]
            tunnel: w473 -> [w801]
            tunnel: w472 -> [w798]
            tunnel: w471 -> [w796]
            tunnel: w468 -> [w792]
            tunnel: [w791] -> w464
            tunnel: w427 -> [w790]
            tunnel: w426 -> [w789]
            tunnel: [w789] -> w425
            tunnel: w423 -> [w788]
            tunnel: w422 -> [w785]
            tunnel: [w873] -> w573
            tunnel: [w872] -> w571
            tunnel: [w871] -> w569
            tunnel: [w870] -> w567
            tunnel: w541 -> [w875]
            tunnel: w539 -> [w874]
            tunnel: w537 -> [w871]
            tunnel: w535 -> [w870]
            tunnel: [w869] -> w565
            tunnel: w533 -> [w869]
            tunnel: [w868] -> w563
            tunnel: w531 -> [w868]
            tunnel: [w867] -> w561
            tunnel: w529 -> [w867]
            tunnel: [w866] -> w559
            tunnel: w527 -> [w866]
            tunnel: [w865] -> w555
            tunnel: w525 -> [w865]
            tunnel: [w864] -> w552
            tunnel: w523 -> [w864]
            tunnel: [w863] -> w549
            tunnel: w521 -> [w863]
            tunnel: [w862] -> w543
            tunnel: w519 -> [w862]
            tunnel: [w861] -> w504
            tunnel: w498 -> [w861]
            tunnel: [w860] -> w493
            tunnel: w492 -> [w860]
            tunnel: [w859] -> w486
            tunnel: w485 -> [w859]
            tunnel: [w858] -> w482
            tunnel: w481 -> [w858]
            tunnel: [w857] -> w476
            tunnel: w475 -> [w857]
            tunnel: [w856] -> w465
            tunnel: w464 -> [w856]
            tunnel: w425 -> [w855]
            tunnel: [w855] -> w424
            tunnel: w573 -> [w896]
            tunnel: [w896] -> w572
            tunnel: w571 -> [w895]
            tunnel: [w895] -> w570
            tunnel: w569 -> [w894]
            tunnel: [w894] -> w568
            tunnel: w567 -> [w893]
            tunnel: [w893] -> w566
            tunnel: w565 -> [w892]
            tunnel: [w892] -> w564
            tunnel: w563 -> [w891]
            tunnel: [w891] -> w562
            tunnel: w561 -> [w890]
            tunnel: [w890] -> w560
            tunnel: w559 -> [w889]
            tunnel: [w889] -> w558
            tunnel: [w888] -> w556
            tunnel: w555 -> [w888]
            tunnel: [w887] -> w553
            tunnel: w552 -> [w887]
            tunnel: [w886] -> w550
            tunnel: w549 -> [w886]
            tunnel: [w885] -> w544
            tunnel: w543 -> [w885]
            tunnel: w504 -> [w884]
            tunnel: [w884] -> w499
            tunnel: [w883] -> w494
            tunnel: w493 -> [w883]
            tunnel: w486 -> [w882]
            tunnel: w482 -> [w881]
            tunnel: [w881] -> w478
            tunnel: [w880] -> w477
            tunnel: w476 -> [w880]
            tunnel: [w879] -> w466
            tunnel: w465 -> [w879]
            tunnel: w424 -> [w877]
            tunnel: w572 -> [w915]
            tunnel: [w920] -> w461
            tunnel: w570 -> [w920]
            tunnel: [w919] -> w459
            tunnel: w568 -> [w919]
            tunnel: [w918] -> w457
            tunnel: w566 -> [w918]
            tunnel: [w916] -> w455
            tunnel: [w914] -> w453
            tunnel: w564 -> [w914]
            tunnel: [w913] -> w451
            tunnel: w562 -> [w913]
            tunnel: [w912] -> w449
            tunnel: w560 -> [w912]
            tunnel: [w911] -> w447
            tunnel: w558 -> [w911]
            tunnel: [w910] -> w445
            tunnel: w556 -> [w910]
            tunnel: [w909] -> w443
            tunnel: w553 -> [w909]
            tunnel: [w908] -> w441
            tunnel: w550 -> [w908]
            tunnel: [w907] -> w439
            tunnel: w544 -> [w907]
            tunnel: [w906] -> w437
            tunnel: w499 -> [w906]
            tunnel: [w905] -> w435
            tunnel: w494 -> [w905]
            tunnel: [w904] -> w433
            tunnel: w478 -> [w904]
            tunnel: [w903] -> w431
            tunnel: w477 -> [w903]
            tunnel: [w902] -> w429
            tunnel: w466 -> [w902]
            tunnel: w461 -> [w941]
            tunnel: [w941] -> w460
            tunnel: w459 -> [w940]
            tunnel: [w940] -> w458
            tunnel: w457 -> [w939]
            tunnel: [w939] -> w456
            tunnel: w455 -> [w938]
            tunnel: [w938] -> w454
            tunnel: w453 -> [w937]
            tunnel: [w937] -> w452
            tunnel: w451 -> [w936]
            tunnel: [w936] -> w450
            tunnel: w449 -> [w935]
            tunnel: [w935] -> w448
            tunnel: w447 -> [w934]
            tunnel: [w934] -> w446
            tunnel: w445 -> [w933]
            tunnel: [w933] -> w444
            tunnel: w443 -> [w924]
            tunnel: [w923] -> w442
            tunnel: w441 -> [w926]
            tunnel: [w925] -> w440
            tunnel: w439 -> [w932]
            tunnel: [w932] -> w438
            tunnel: w437 -> [w931]
            tunnel: [w931] -> w436
            tunnel: w435 -> [w930]
            tunnel: [w930] -> w434
            tunnel: w433 -> [w929]
            tunnel: [w929] -> w432
            tunnel: w431 -> [w928]
            tunnel: [w928] -> w430
            tunnel: w429 -> [w927]
            tunnel: [w927] -> w428
            tunnel: w460 -> [w961]
            tunnel: w458 -> [w960]
            tunnel: w456 -> [w959]
            tunnel: w454 -> [w963]
            tunnel: w452 -> [w956]
            tunnel: w450 -> [w955]
            tunnel: [w964] -> w588
            tunnel: [w962] -> w587
            tunnel: [w958] -> w586
            tunnel: [w957] -> w585
            tunnel: [w956] -> w584
            tunnel: [w955] -> w583
            tunnel: [w954] -> w581
            tunnel: w448 -> [w954]
            tunnel: [w953] -> w578
            tunnel: w446 -> [w953]
            tunnel: [w952] -> w557
            tunnel: w444 -> [w952]
            tunnel: [w951] -> w554
            tunnel: w442 -> [w951]
            tunnel: [w950] -> w551
            tunnel: w440 -> [w950]
            tunnel: [w949] -> w545
            tunnel: w438 -> [w949]
            tunnel: [w948] -> w500
            tunnel: w436 -> [w948]
            tunnel: w434 -> [w947]
            tunnel: [w947] -> w490
            tunnel: [w946] -> w483
            tunnel: w432 -> [w946]
            tunnel: w430 -> [w943]
            tunnel: [w942] -> w467
            tunnel: w428 -> [w942]
            tunnel: [w1006] -> w589
            tunnel: [w1004] -> w590
            tunnel: [w1024] -> w594
            tunnel: [w1025] -> w595
            tunnel: [w1026] -> w598
            tunnel: [w1027] -> w599
            tunnel: w588 -> [w1027]
            tunnel: w587 -> [w1026]
            tunnel: w586 -> [w1025]
            tunnel: w585 -> [w1024]
            tunnel: w584 -> [w1005]
            tunnel: w583 -> [w1007]
            tunnel: [w1023] -> w582
            tunnel: w581 -> [w1023]
            tunnel: [w1022] -> w579
            tunnel: w578 -> [w1022]
            tunnel: w557 -> [w1018]
            tunnel: w554 -> [w1001]
            tunnel: w551 -> [w1002]
            tunnel: [w1019] -> w546
            tunnel: w545 -> [w1019]
            tunnel: [w994] -> w501
            tunnel: w500 -> [w996]
            tunnel: [w995] -> w491
            tunnel: w490 -> [w997]
            tunnel: [w1001] -> w489
            tunnel: [w1002] -> w488
            tunnel: [w1010] -> w484
            tunnel: w483 -> [w1009]
            tunnel: [w1009] -> w479
            tunnel: w467 -> [w1003]
            tunnel: [w1003] -> w463
            frame #0 {
              # "Current frame (0 indexed)"
              # "Current channel (0 indexed)"
              # "Calculate current channel"
              # "Pre exposure tasks:"
              # "Move z piezo"
              n107 = local read "#z-planes"() -> (w618:i16)
              n108 = local read "Z move"() -> (w615:bool)
              n109 = local read "SIM Frames"() -> (w604:i16)
              n110 = local read "#Channels"() -> (w607:i16)
              n111 = Greater?(x=w618, y=i16 1) -> (0:w616:bool)
              n112 = And(x=w615, y=w616) -> (x .and. y?=w614:bool)
              n113 = Divide(x=w609, y=w604) -> (x/y=w610:dbl)
              n114 = Round Toward -Infinity(1:w610) -> (0:w608:dbl)
              n115 = Quotient & Remainder(x=w608, y=w607) -> (x-y*floor(x/y)=w605:dbl)  [unwired: 1 out]
              n116 = case shown="False" w614 {
                tunnel: w602 -> [w634 w635]
                tunnel: [w634 w648] -> w613
                tunnel: w612 -> [w633 w641]
                tunnel: [w633 w640] -> w611
                frame False {
                  n117 = local read "z0 (um)"() -> (w632:dbl)
                  n118 = local write "Current z-position (um)"(w632) -> ()
                }
                frame True {
                  n119 = local read "Current z #"() -> (w636:i16)
                  n120 = local read "z0 (um)"() -> (w646:dbl)
                  n121 = local read "#z-planes"() -> (w649:i16)
                  n122 = local read "z-step (um)"() -> (w644:dbl)
                  n123 = Decrement(x=w636) -> (x-1=w637:i16)
                  n124 = Greater?(x=w636, y=w649) -> (0:w645:bool)
                  n125 = Multiply(x=w637, y=w644) -> (x*y=w643:dbl)
                  n126 = Add(x=w646, y=w643) -> (x+y=w647:dbl)
                  n127 = Select(t=w646, s=w645, f=w647) -> (s? t:f=w638:dbl)
                  n128 = local read "Z-move method"() -> (w642:u16)
                  n129 = local write "Current z-position (um)"(w638) -> ()
                  n130 = case shown="True" w645 {
                    frame False {
                    }
                    frame True {
                      n131 = local write "Current z #"(i16 1 ("z #")) -> ()
                    }
                  }
                  n132 = call "WriteZ.vi"("new-z (um)"=w638, "Method"=w642, "error in (no error)"=w635, "ASI VISA resource name"=w641) -> ("error out"=w648:errorcluster, "V"=w639:dbl, "ASI VISA resource name OUT"=w640:refnum<visa-resource-name>)  [unwired: 5 in]
                  n133 = local write "Current piezo position (V)"(w639) -> ()
                  n134 = local write "Z move"(FALSE) -> ()
                }
              }
              n135 = To Unsigned Byte Integer(number=w605) -> (unsigned 8bit integer=w606:u8)
            }
            frame #1 {
              # "Final frame for this z-position?"
              # "Pre exposure tasks:"
              # "Set laser, filter and pockels voltage"
              n136 = local read "TIRF Mode N"() -> (w657:T3)
              n137 = local read "Optosplit"() -> (w654:bool)
              n138 = local read "Widefield?"() -> (w655:bool)
              n139 = local read "Voltages:"() -> (w669:dbl[][])
              n140 = call "Channel ID to Wave ID.vi"("Ch N"=w681, "Channel ID"=w653) -> ("Wave ID"=w659:i16)  [unwired: 9 in]
              n141 = call "Channel ID to Mode ID.vi"("TIRF Mode N"=w657, "Widefield mode?"=w655, "Channel ID"=w653) -> ("Mode ID"=w656:i8)  [unwired: 8 in]
              n142 = case shown="False" w654 {
                tunnel: w683 -> [w698 w775]
                tunnel: w682 -> [w697 w773]
                tunnel: [w696 w774] -> w680
                tunnel: [w695 w772] -> w679
                tunnel: w678 -> [w694 w768]
                tunnel: w677 -> [w693 w763]
                tunnel: [w692 w765] -> w676
                tunnel: [w691 w764] -> w661
                tunnel: w659 -> [w690 _]
                frame False {
                  n143 = case shown="0, Default" w690 {
                    tunnel: w698 -> [w712 w730 w752]
                    tunnel: w697 -> [w711 w729 w751]
                    tunnel: [w710 w732 w750] -> w696
                    tunnel: [w709 w731 w749] -> w695
                    tunnel: w694 -> [w707 w724 w745]
                    tunnel: w693 -> [w708 w723 w746]
                    tunnel: [w706 w725 w744] -> w692
                    tunnel: [w705 w726 w743] -> w691
                    frame 0, Default {
                      w699 = bool[] [TRUE, FALSE, FALSE] ("data")
                      # "Wavelength 0: 488nm"
                      n144 = local read "Current filter"() -> (w703:string)
                      n145 = local read "Filter 488"() -> (w702:i8)
                      n146 = call-poly <vilib>:"DAQmx Write.vi"("task/channels in"=w712, "data"=w699, "error in"=w711) -> ("task out"=w710:refnum<k21>, "error out"=w709:errorcluster)  [unwired: 10 in, 1 out]
                      n147 = Number To Decimal String(number=w702) -> (decimal integer string=w701:string)  [unwired: 1 in]
                      n148 = Equal?(x=w701, y=w703) -> (x = y?=w704:bool)
                      n149 = case shown="False" w704 {
                        tunnel: w708 -> [w716 w717]
                        tunnel: w707 -> [w714 w718]
                        tunnel: w701 -> [w713 _]
                        tunnel: [w714 w718] -> w706
                        tunnel: [w715 w717] -> w705
                        frame False {
                          n150 = call "Change_filter.vi"("error in"=w716, "filter number"=w713, "VISA resource name"=w714) -> ("error out"=w715:errorcluster)  [unwired: 7 in, 1 out]
                          n151 = local write "Current filter"(w713) -> ()
                        }
                        frame True {
                        }
                      }
                      n152 = Array To Cluster(array=w699) -> (cluster=w700:T12)
                      n153 = local write "Laser Cluster"(w700) -> ()
                    }
                    frame 1 {
                      w719 = bool[] [FALSE, FALSE, TRUE] ("data")
                      # "Wavelength 2: 561 nm"
                      n154 = local read "Filter 561"() -> (w722:i8)
                      n155 = local read "Current filter"() -> (w727:string)
                      n156 = Number To Decimal String(number=w722) -> (decimal integer string=w721:string)  [unwired: 1 in]
                      n157 = Equal?(x=w721, y=w727) -> (x = y?=w728:bool)
                      n158 = case shown="False" w728 {
                        tunnel: w723 -> [w736 w737]
                        tunnel: w724 -> [w734 w738]
                        tunnel: w721 -> [w733 _]
                        tunnel: [w734 w738] -> w725
                        tunnel: [w735 w737] -> w726
                        frame False {
                          n159 = call "Change_filter.vi"("error in"=w736, "filter number"=w733, "VISA resource name"=w734) -> ("error out"=w735:errorcluster)  [unwired: 7 in, 1 out]
                          n160 = local write "Current filter"(w733) -> ()
                        }
                        frame True {
                        }
                      }
                      n161 = call-poly <vilib>:"DAQmx Write.vi"("task/channels in"=w730, "data"=w719, "error in"=w729) -> ("task out"=w732:refnum<k21>, "error out"=w731:errorcluster)  [unwired: 10 in, 1 out]
                      n162 = Array To Cluster(array=w719) -> (cluster=w720:T12)
                      n163 = local write "Laser Cluster"(w720) -> ()
                    }
                    frame 2 {
                      w739 = bool[] [FALSE, TRUE, FALSE] ("data")
                      # "Wavelength 1: 640nm"
                      n164 = local read "Filter 640"() -> (w742:i8)
                      n165 = local read "Current filter"() -> (w747:string)
                      n166 = Number To Decimal String(number=w742) -> (decimal integer string=w741:string)  [unwired: 1 in]
                      n167 = Equal?(x=w741, y=w747) -> (x = y?=w748:bool)
                      n168 = call-poly <vilib>:"DAQmx Write.vi"("task/channels in"=w752, "data"=w739, "error in"=w751) -> ("task out"=w750:refnum<k21>, "error out"=w749:errorcluster)  [unwired: 10 in, 1 out]
                      n169 = case shown="False" w748 {
                        tunnel: w746 -> [w756 w757]
                        tunnel: w745 -> [w754 w758]
                        tunnel: w741 -> [w753 _]
                        tunnel: [w754 w758] -> w744
                        tunnel: [w755 w757] -> w743
                        frame False {
                          n170 = call "Change_filter.vi"("error in"=w756, "filter number"=w753, "VISA resource name"=w754) -> ("error out"=w755:errorcluster)  [unwired: 7 in, 1 out]
                          n171 = local write "Current filter"(w753) -> ()
                        }
                        frame True {
                        }
                      }
                      n172 = Array To Cluster(array=w739) -> (cluster=w740:T12)
                      n173 = local write "Laser Cluster"(w740) -> ()
                    }
                  }
                }
                frame True {
                  n174 = local read "Current filter"() -> (w767:string)
                  n175 = local read "Filter Optosplit"() -> (w762:i8)
                  n176 = local read "488-OS"() -> (w769:bool)
                  n177 = local read "640-OS"() -> (w771:bool)
                  n178 = local read "561-OS"() -> (w770:bool)
                  n179 = Number To Decimal String(number=w762) -> (decimal integer string=w761:string)  [unwired: 1 in]
                  n180 = Equal?(x=w761, y=w767) -> (x = y?=w766:bool)
                  n181 = Build Array(w769, w771, w770) -> (w760:bool[])
                  n182 = case shown="False" w766 {
                    tunnel: w768 -> [w780 w782]
                    tunnel: [w779 w782] -> w765
                    tunnel: w761 -> [w778 _]
                    tunnel: [w777 w781] -> w764
                    tunnel: w763 -> [w776 w781]
                    frame False {
                      n183 = local write "Current filter"(w778) -> ()
                      n184 = call "Change_filter.vi"("error in"=w776, "filter number"=w778, "VISA resource name"=w780) -> ("error out"=w777:errorcluster, "VISA resource name out"=w779:refnum<visa-resource-name>)  [unwired: 7 in]
                    }
                    frame True {
                    }
                  }
                  n185 = Array To Cluster(array=w760) -> (cluster=w759:cluster{"[0]":bool, "[1]":bool, "[2]":bool})
                  n186 = call-poly <vilib>:"DAQmx Write.vi"("task/channels in"=w775, "data"=w760, "error in"=w773) -> ("task out"=w774:refnum<k21>, "error out"=w772:errorcluster)  [unwired: 10 in, 1 out]
                  n187 = local write "Laser Cluster"(w759) -> ()
                }
              }
              n188 = call "Select Voltage From Wavelength.vi"("Voltages"=w669, "Mode"=w656, "Wavelength"=w659, "SIM Frame"=w652) -> ("Voltage out"=w668:dbl)  [unwired: 7 in]
              n189 = local read "SIM Frames"() -> (w665:i16)
              n190 = local read "#Channels"() -> (w666:i16)
              n191 = call-poly <vilib>:"DAQmx Write.vi"("task/channels in"=w673, "data"=w668, "error in"=w671) -> ("task out"=w672:refnum<k21>, "error out"=w670:errorcluster)  [unwired: 10 in, 1 out]
              n192 = Increment(x=w652) -> (x+1=w660:i32)
              n193 = Multiply(x=w666, y=w665) -> (x*y=w664:i16)
              n194 = Quotient & Remainder(x=w660, y=w664) -> (x-y*floor(x/y)=w663:i32)  [unwired: 1 out]
              n195 = Equal?(x=w663, y=0) -> (x = y?=w667:bool)
            }
            frame #2 {
              # "First frame of this channel?"
              # "Set SLM for this channel"
              # "Pre exposure tasks:"
              # "Offset piezo for this channel"
              n196 = local read "Manual SLM mode"() -> (w797:bool)
              n197 = case shown="False" w797 {
                tunnel: w798 -> [w835 _]
                tunnel: [w834 w842] -> w794
                tunnel: w796 -> [w833 _]
                tunnel: w790 -> [w832 _]
                frame False {
                  n198 = case shown="True" w832 {
                    tunnel: w835 -> [w838 _]
                    tunnel: [w837 w839] -> w834
                    tunnel: w833 -> [w836 w841]
                    frame False {
                      n199 = call "RO from WL and mode.vi"("Mode"=w836, "Wavelength"=w838) -> ("SLM pattern"=w837:u8)  [unwired: 9 in]
                    }
                    frame True {
                      n200 = call "RO from WL and mode.vi"("Mode"=w841, "Wavelength"=u8 1) -> ("SLM pattern"=w839:u8)  [unwired: 9 in]
                    }
                  }
                }
                frame True {
                  n201 = local read "RO"() -> (w842:u8)
                }
              }
              n202 = local read "use z offset"() -> (w805:bool)
              n203 = local read "Current RO"() -> (w795:u8)
              n204 = local read "SIM Frames"() -> (w783:i16)
              n205 = Not Equal?(x=w794, y=w795) -> (x != y?=w793:bool)
              n206 = Quotient & Remainder(x=w785, y=w783) -> (x-y*floor(x/y)=w786:i32)  [unwired: 1 out]
              n207 = case shown="True" w793 {
                tunnel: w794 -> [_ w825]
                tunnel: w792 -> [w820 w823]
                tunnel: [w820 w821] -> w791
                frame False {
                }
                frame True {
                  n208 = call <userlib>:"set Selected RO.vi"("error in (no error)"=w823, "runningOrder"=w825) -> ("error out"=w822:errorcluster, "function return"=w824:i16)  [unwired: 8 in]
                  n209 = case shown="0, Default" w824 {
                    tunnel: w822 -> [w828 w831]
                    tunnel: [w826 w831] -> w821
                    frame 0, Default {
                      n210 = call <userlib>:"get Activation State.vi"("error in (no error)"=w828) -> ("error out"=w827:errorcluster, "String"=w830:string)  [unwired: 7 in, 2 out]
                      n211 = local write "SLM State"(w830) -> ()
                      n212 = call <userlib>:"get Selected RO.vi"("error in (no error)"=w827) -> ("error out"=w826:errorcluster, "selectedRO"=w829:u8)  [unwired: 8 in, 1 out]
                      n213 = local write "Current RO"(w829) -> ()
                    }
                    frame 1 {
                    }
                  }
                }
              }
              n214 = Equal?(x=w786, y=0) -> (x = y?=w784:bool)
              n215 = And(x=w805, y=w784) -> (x .and. y?=w808:bool)
              n216 = case shown="True" w808 {
                tunnel: w807 -> [w844 w851]
                tunnel: [w844 w850] -> w806
                tunnel: w804 -> [w843 w848]
                tunnel: [w843 w847] -> w803
                tunnel: w788 -> [_ w845]
                frame False {
                }
                frame True {
                  n217 = local read "Z offset (um)"() -> (w853:dbl[])
                  n218 = local read "Current z-position (um)"() -> (w854:dbl)
                  n219 = local read "Z-move method"() -> (w849:u16)
                  n220 = Index Array(array=w853, index=w845) -> (element=w852:dbl)
                  n221 = Add(x=w854, y=w852) -> (x+y=w846:dbl)
                  n222 = call "WriteZ.vi"("new-z (um)"=w846, "Method"=w849, "error in (no error)"=w851, "ASI VISA resource name"=w848) -> ("error out"=w850:errorcluster, "ASI VISA resource name OUT"=w847:refnum<visa-resource-name>)  [unwired: 5 in, 1 out]
                }
              }
            }
            frame #3 {
              # "Start camera exposure"
              n223 = call-poly <vilib>:"DAQmx Write.vi"("task/channels in"=w875, "data"=TRUE, "error in"=w874) -> ("task out"=w873:refnum<k21>, "error out"=w872:errorcluster)  [unwired: 10 in, 1 out]
            }
            frame #4 {
              # "Expose camera"
              n224 = case shown="True" w877 {
                tunnel: w882 -> [w898 _]
                tunnel: [w897 w900] -> w878
                frame False {
                  n225 = local read "Exposure times N"() -> (w899:dbl[])
                  n226 = Index Array(array=w899, index=w898) -> (element=w897:dbl)
                }
                frame True {
                  n227 = local read "Exp OS"() -> (w901:string)
                  n228 = Decimal String To Number(string=w901) -> (number=w900:i32)  [unwired: 2 in, 1 out]
                }
              }
              n229 = Wait (ms)(milliseconds to wait=w878) -> ()  [unwired: 1 out]
            }
            frame #5 {
              # "End camera exposure"
              n230 = call-poly <vilib>:"DAQmx Write.vi"("task/channels in"=w915, "data"=FALSE) -> ("task out"=w916:refnum<k21>)  [unwired: 11 in, 2 out]
            }
            frame #6 {
              w921 = bool[] [FALSE, FALSE, FALSE] ("data")
              # "Switch off the laser"
              n231 = Array To Cluster(array=w921) -> (cluster=w922:T12)
              n232 = call-poly <vilib>:"DAQmx Write.vi"("task/channels in"=w924, "data"=w921, "error in"=w926) -> ("task out"=w923:refnum<k21>, "error out"=w925:errorcluster)  [unwired: 10 in, 1 out]
              n233 = local write "Laser Cluster"(w922) -> ()
            }
            frame #7 {
              # "Current frame + 1"
              # "I think that we are correct not to wait for the \ntrigger ready on the very last frame. mjf74"
              n234 = local read "Total\nFrames"() -> (w944:i16)
              n235 = Equal?(x=w944, y=w943) -> (x = y?=w945:bool)
              n236 = case shown="False" w945 {
                tunnel: [w972 w985] -> w964
                tunnel: w963 -> [w971 w985]
                tunnel: [w970 w984] -> w962
                tunnel: w961 -> [w969 w984]
                tunnel: w960 -> [w968 w983]
                tunnel: w959 -> [w967 w982]
                tunnel: [w966 w982] -> w958
                tunnel: [w965 w983] -> w957
                frame False {
                  # "Wait until Trigger Ready received"
                  n237 = while {
                    tunnel: [w981] -> w972
                    tunnel: w971 -> [w981]
                    tunnel: [w980] -> w970
                    tunnel: w969 -> [w980]
                    tunnel: w968 -> [w979]
                    tunnel: w967 -> [w978]
                    tunnel: [w977] -> w966
                    tunnel: [w976] -> w965
                    stop <- w973 stop-if-true
                    n238 = local read "stop"() -> (w975:bool)
                    n239 = call-poly <vilib>:"DAQmx Read.vi"("task/channels in"=w979, "error in"=w978) -> ("task out"=w976:refnum<k21>, "data"=w974:bool, "error out"=w977:errorcluster)  [unwired: 11 in]
                    n240 = Or(x=w974, y=w975) -> (x .or. y?=w973:bool)
                  }
                }
                frame True {
                }
              }
            }
            frame #8 {
              # "Write 0V to Pockels"
              # "Post exposure tasks"
              n241 = local read "SIM Frames"() -> (w1017:i16)
              n242 = local read "#Channels"() -> (w1016:i16)
              n243 = local read "#bookmarks"() -> (w989:i16)
              n244 = local read "#z-planes"() -> (w1014:i16)
              n245 = local read "Current \nFrame"() -> (w999:i32)
              n246 = Multiply(x=w1017, y=w1016) -> (x*y=w1015:i16)
              n247 = Not Equal To 0?(x=w989) -> (x != 0?=w986:bool)
              n248 = Multiply(x=w1014, y=w1015) -> (x*y=w992:i16)
              n249 = Select(t=w989, s=w986, f=i16 1 ("t")) -> (s? t:f=w991:i16)
              n250 = Quotient & Remainder(x=w999, y=w992) -> (x-y*floor(x/y)=w1013:i32)  [unwired: 1 out]
              n251 = Multiply(x=w991, y=w992) -> (x*y=w1000:i16)
              n252 = Quotient & Remainder(x=w999, y=w1000) -> (x-y*floor(x/y)=w998:i32)  [unwired: 1 out]
              n253 = Equal To 0?(x=w1013) -> (x = 0?=w988:bool)
              n254 = And(x=w988, y=w986) -> (x .and. y?=w987:bool)
              n255 = Equal To 0?(x=w998) -> (x = 0?=w993:bool)
              n256 = case shown="True" w987 {
                tunnel: w997 -> [w1029 w1037]
                tunnel: w996 -> [w1028 w1036]
                tunnel: [w1029 w1035] -> w995
                tunnel: [w1028 w1034] -> w994
                tunnel: w993 -> [_ w1030]
                frame False {
                }
                frame True {
                  n257 = flat-sequence {
                    tunnel: w1036 -> [w1040]
                    tunnel: w1037 -> [w1041]
                    tunnel: [w1041] -> w1033
                    tunnel: [w1040] -> w1032
                    tunnel: [w1039] -> w1031
                    tunnel: w1030 -> [w1038]
                    tunnel: [w1047] -> w1035
                    tunnel: [w1046] -> w1034
                    tunnel: w1033 -> [w1049]
                    tunnel: w1032 -> [w1048]
                    tunnel: w1031 -> [w1045]
                    frame #0 {
                      n258 = case shown="True" w1038 {
                        tunnel: [w1042 w1044] -> w1039
                        frame False {
                          n259 = local read "Current bookmark"() -> (w1043:i32)
                          n260 = Increment(x=w1043) -> (x+1=w1042:i32)
                          n261 = local write "Current bookmark"(w1042) -> ()
                        }
                        frame True {
                          w1044 = 0.0 ("Current bookmark")
                          n262 = local write "Current bookmark"(w1044) -> ()
                        }
                      }
                    }
                    frame #1 {
                      w1057 = u16 1 items=["X", "Y", "Z"] ("Axis")
                      w1064 = u16 0 items=["X", "Y", "Z"] ("Axis")
                      n263 = property on="Bookmark List" class="MCListbox (strict)"() -> ("ItemNames"=w1061:string[][])  [unwired: 2 in, 2 out]
                      n264 = Index Array(array=w1061, index (row)=w1045, index (col)=1 ("disabled index (col)")) -> (element=w1060:string)
                      n265 = Index Array(array=w1061, index (row)=w1045, index (col)=2 ("disabled index (col)")) -> (element=w1055:string)
                      n266 = Decimal String To Number(string=w1055) -> (number=w1050:i32)  [unwired: 2 in, 1 out]
                      n267 = Decimal String To Number(string=w1060) -> (number=w1053:i32)  [unwired: 2 in, 1 out]
                      n268 = To Double Precision Float(number=w1053) -> (double precision float=w1052:dbl)
                      n269 = call "ASI_move_serial.vi"("Position/distance (um)"=w1052, "error in"=w1048, "Relative?"=FALSE, "Axis"=w1064, "VISA resource name"=w1049) -> ("error out"=w1054:errorcluster, "VISA resource name out"=w1058:refnum<visa-resource-name>)  [unwired: 2 in]
                      n270 = To Double Precision Float(number=w1050) -> (double precision float=w1051:dbl)
                      n271 = call "ASI_move_serial.vi"("Position/distance (um)"=w1051, "error in"=w1054, "Relative?"=FALSE, "Axis"=w1057, "VISA resource name"=w1058) -> ("error out"=w1046:errorcluster, "VISA resource name out"=w1047:refnum<visa-resource-name>)  [unwired: 2 in]
                    }
                  }
                }
              }
              n272 = local read "t-interval"() -> (w1021:u32)
              n273 = case shown="True" w1018 {
                frame False {
                }
                frame True {
                  # "if it's the final frame at this z, \nmove the z position for the next frame"
                  n274 = local read "Current z #"() -> (w1066:i16)
                  n275 = Increment(x=w1066) -> (x+1=w1065:i16)
                  n276 = local write "Current z #"(w1065) -> ()
                  n277 = local write "Z move"(TRUE) -> ()
                }
              }
              n278 = call-poly <vilib>:"DAQmx Write.vi"("task/channels in"=w1005, "data"=0.0, "error in"=w1007) -> ("task out"=w1004:refnum<k21>, "error out"=w1006:errorcluster)  [unwired: 10 in, 1 out]
              n279 = Not Equal To 0?(x=w1021) -> (x != 0?=w1020:bool)
              n280 = And(x=w1018, y=w1020) -> (x .and. y?=w1012:bool)
              n281 = And(x=w1012, y=w993) -> (x .and. y?=w1011:bool)
              n282 = case shown="True" w1011 {
                tunnel: w1021 -> [_ w1068]
                frame False {
                }
                frame True {
                  # "If it's the final frame at this t,\nwait for the required interval"
                  # "Wait for requested duration"
                  n283 = local read "Int unit"() -> (w1069:enum16{"ms", "s", "min"})
                  n284 = call "Wait Interval.vi"("Interval unit"=w1069, "Interval"=w1068) -> ("Wait"=w1070:u32)  [unwired: 9 in]
                  n285 = Wait (ms)(milliseconds to wait=w1070) -> ()  [unwired: 1 out]
                }
              }
              n286 = local read "stop"() -> (w1010:bool)
            }
          }
          n287 = Increment(x=w593) -> (x+1=w420:i32)
          "Current \nFrame" <- w420
        }
        n288 = call-poly <vilib>:"DAQmx Write.vi"("task/channels in"=w337, "data"=FALSE, "error in"=w335) -> ("task out"=w336:refnum<k21>, "error out"=w334:errorcluster)  [unwired: 10 in, 1 out]
        n289 = flat-sequence {
          tunnel: w325 -> [w412]
          tunnel: w324 -> [w411]
          tunnel: [w407] -> w320
          tunnel: [w403] -> w301
          frame #0 {
            # "Re-enable joystick"
            # "Piezo position"
            n290 = local read "z0 (um)"() -> (w402:dbl)
            n291 = local read "Z-move method"() -> (w406:u16)
            n292 = local write "Current z-position (um)"(w402) -> ()
            n293 = call "WriteZ.vi"("new-z (um)"=w402, "Method"=w406, "error in (no error)"=w412, "ASI VISA resource name"=w411) -> ("error out"=w408:errorcluster, "V"=w405:dbl, "ASI VISA resource name OUT"=w409:refnum<visa-resource-name>)  [unwired: 5 in]
            n294 = local write "Current bookmark"(0.0 ("Current bookmark")) -> ()
            n295 = local write "Current piezo position (V)"(w405) -> ()
            n296 = call "ASI_Disable_Enable_Controls.vi"("Enable Z"=TRUE ("Disable Z"), "error in"=w408, "Enable XY"=TRUE ("Disable Z"), "VISA resource name"=w409) -> ("error out"=w407:errorcluster, "VISA resource name out"=w403:refnum<visa-resource-name>)
          }
        }
        n297 = flat-sequence {
          tunnel: [w367] -> w289
          tunnel: w288 -> [w363]
          tunnel: [w362] -> w287
          tunnel: w286 -> [w361]
          frame #0 {
            # "Post to Labstep"
            n298 = local read "Exposure times N"() -> (w371:dbl[])
            n299 = local read "TIRF Mode N"() -> (w370:T3)
            n300 = local read "Total\nFrames"() -> (w377:i16)
            n301 = local read "#bookmarks"() -> (w373:i16)
            n302 = local read "z-step (um)"() -> (w366:dbl)
            n303 = local read "#Channels"() -> (w376:i16)
            n304 = property on="Int unit" class="Enum (strict)"() -> ("RingText.Text"=w364:string)  [unwired: 2 in, 2 out]
            n305 = local read "Widefield?"() -> (w368:bool)
            n306 = local read "#t-frames"() -> (w375:i16)
            n307 = local read "#z-planes"() -> (w374:i16)
            n308 = local read "Optosplit"() -> (w369:bool)
            n309 = local read "t-interval"() -> (w365:u32)
            n310 = local read "Ch N"() -> (w372:T7)
            n311 = local read "User"() -> (w378:string)
            n312 = Bundle(cluster=T10 {"User"="", "Total\nFrames"=0, "#Channels"=0, "#t-frames"=0, "#z-planes"=0, "#bookmarks"=0, "Ch N"={"Ch 0"=enum."Radio Selection 1", "Ch 1"=enum."Radio Selection 1", "Ch 2"=enum."Radio Selection 1"}, "Exposure times N"=[], "TIRF Mode N"={"Boolean 1"=FALSE, "Boolean 2"=FALSE, "Boolean 3"=FALSE}, "Optosplit"=FALSE, "Widefield?"=FALSE, "t-interval"=0, "RingText.Text"="", "z-step (um)"=0.0, 0}, "User"=w378, "Total\nFrames"=w377, "#Channels"=w376, "#t-frames"=w375, "#z-planes"=w374, "#bookmarks"=w373, "Ch N"=w372, "Exposure times N"=w371, "TIRF Mode N"=w370, "Optosplit"=w369, "Widefield?"=w368, "t-interval"=w365, "RingText.Text"=w364, "z-step (um)"=w366, w361) -> (w359:T10)
            n313 = call "Gather image parameters.vi"("error in"=w363, "Acq params"=w359) -> ("error out"=w362:errorcluster, "Acqusition string"=w367:string)  [unwired: 8 in]
          }
        }
        n314 = VISA Close(VISA resource name=w339, error in (no error)=w309) -> (error out=w308:errorcluster)
        n315 = Merge Errors(w353, w352, w307, w308, w317) -> (w288:errorcluster)
        n316 = Unbundle By Name(w288) -> ("status"=w316:bool)
        n317 = local read "Labstep API_Key"() -> (w291:string)
        n318 = flat-sequence {
          tunnel: [w415] -> w315
          tunnel: w307 -> [w415]
          tunnel: [w414] -> w314
          tunnel: w306 -> [w414]
          frame #0 {
            w416 = FALSE ("Z move")
            # "Reset buttons"
            n319 = local write "Z move"(w416) -> ()
            n320 = local write "Acquire"(w416) -> ()
            n321 = property on="Acquire" class="Bool (strict)"("DisabledEnum"=T11."Enabled" ("Disabled")) -> ()  [unwired: 2 in, 2 out]
          }
        }
        n322 = call "Add post to experiment.vi"("API Key"=w291, "error in"=w287, "Thread ID"=w285, "Post contents"=w289) -> ()  [unwired: 7 in, 1 out]
      }
      event "Optosplit": Value Change {
        w1077 = 2.0 ("f")
        w1076 = 0.0 ("t")
        n323 = event-data() -> ("NewVal"=w1072:bool)  [unwired: 1 in]
        n324 = Select(t=w1077, s=w1072, f=w1076) -> (s? t:f=w1074:dbl)
        n325 = Select(t=w1076, s=w1072, f=w1077) -> (s? t:f=w1075:dbl)
        n326 = property on="Exp 1" class="DigNum (strict)"("DisabledEnum"=w1074) -> ()  [unwired: 2 in, 2 out]
        n327 = property on="Exp 2" class="DigNum (strict)"("DisabledEnum"=w1074) -> ()  [unwired: 2 in, 2 out]
        n328 = property on="Live OS Channel Cluster" class="Clust (strict)"("Visible"=w1072) -> ()  [unwired: 2 in, 2 out]
        n329 = property on="#Channels" class="DigNum (strict)"("Val(Sgnl)"=i16 1 ("#Channels")) -> ()  [unwired: 2 in, 2 out]
        n330 = property on="Ch2 TIRF" class="Bool (strict)"("DisabledEnum"=w1074) -> ()  [unwired: 2 in, 2 out]
        n331 = property on="Ch 3" class="RadioBtnsControl (strict)"("DisabledEnum"=w1074) -> ()  [unwired: 2 in, 2 out]
        n332 = property on="Exp 0" class="DigNum (strict)"("DisabledEnum"=w1074) -> ()  [unwired: 2 in, 2 out]
        n333 = property on="Ch1 TIRF" class="Bool (strict)"("DisabledEnum"=w1074) -> ()  [unwired: 2 in, 2 out]
        n334 = property on="Ch3 TIRF" class="Bool (strict)"("DisabledEnum"=w1074) -> ()  [unwired: 2 in, 2 out]
        n335 = property on="Ch 2" class="RadioBtnsControl (strict)"("DisabledEnum"=w1074) -> ()  [unwired: 2 in, 2 out]
        n336 = property on="488-OS" class="Bool (strict)"("DisabledEnum"=w1075) -> ()  [unwired: 2 in, 2 out]
        n337 = property on="Ch 1" class="RadioBtnsControl (strict)"("DisabledEnum"=w1074) -> ()  [unwired: 2 in, 2 out]
        n338 = property on="561-OS" class="Bool (strict)"("DisabledEnum"=w1075) -> ()  [unwired: 2 in, 2 out]
        n339 = property on="640-OS" class="Bool (strict)"("DisabledEnum"=w1075) -> ()  [unwired: 2 in, 2 out]
        n340 = property on="Exp OS" class="Str"("DisabledEnum"=w1075) -> ()  [unwired: 2 in, 2 out]
      }
      event "Sweep": Value Change {
        n341 = event-data() -> ()  [unwired: 1 in, 4 out]
        n342 = local read "Sweep Pattern"() -> (w1095:u8)
        n343 = case shown="21..23, Default" w1095 {
          tunnel: [9 12 15] -> w1094
          frame 21..23, Default {
          }
          frame 24..26 {
          }
          frame 27..29 {
          }
        }
        n344 = call-poly <vilib>:"DAQmx Write.vi"("task/channels in"=w1138, "data"=FALSE, "error in"=w1137) -> ("task out"=w1139:refnum<k21>, "error out"=w1141:errorcluster)  [unwired: 10 in, 1 out]
        n345 = flat-sequence {
          tunnel: [w1168] -> w1142
          tunnel: w1141 -> [w1168]
          tunnel: [w1167] -> w1140
          tunnel: w1139 -> [w1167]
          frame #0 {
            n346 = Wait (ms)(milliseconds to wait=u32 100) -> ()  [unwired: 1 out]
          }
        }
        n347 = local write "Step index:"(u16 0 ("V step")) -> ()
        n348 = call-poly <vilib>:"DAQmx Write.vi"("task/channels in"=w1140, "data"=TRUE, "error in"=w1142) -> ("task out"=w1125:refnum<k21>, "error out"=w1124:errorcluster)  [unwired: 10 in, 1 out]
        n349 = local read "V. steps"() -> (w1146:i16)
        n350 = Multiply(x=w1146, y=w1094) -> (x*y=w1145:i32)
        n351 = for {
          N: w1145 -> [w1171]
          tunnel: w1136 -> [w1291]
          tunnel: w1135 -> [w1290]
          tunnel: w1134 -> [w1289]
          tunnel: w1133 -> [w1288]
          tunnel: w1132 -> [w1287]
          tunnel: w1131 -> [w1286]
          tunnel: w1130 -> [w1284]
          tunnel: w1129 -> [w1282]
          tunnel: w1128 -> [w1280]
          tunnel: w1127 -> [w1278]
          tunnel: w1125 -> [w1260]
          tunnel: w1124 -> [w1256]
          tunnel: [w1220] -> w1123
          tunnel: [w1221] -> w1122
          tunnel: [w1243] -> w1115
          tunnel: [w1242] -> w1117
          tunnel: [w1241] -> w1119
          tunnel: [w1240] -> w1118
          tunnel: [w1235] -> w1116
          tunnel: [w1234] -> w1099
          tunnel: [w1233] -> w1102
          tunnel: [w1232] -> w1103
          tunnel: [w1223] -> w1111
          tunnel: [w1222] -> w1108
          tunnel: w1107 -> [w1206]
          tunnel: [w1200] -> w1106
          tunnel: w1094 -> [w1169]
          i -> [w1173]
          n352 = flat-sequence {
            tunnel: w1256 -> [w1299]
            tunnel: w1260 -> [w1300]
            tunnel: w1278 -> [w1301]
            tunnel: w1280 -> [w1302]
            tunnel: w1282 -> [w1303]
            tunnel: w1284 -> [w1304]
            tunnel: w1286 -> [w1305]
            tunnel: w1287 -> [w1306]
            tunnel: w1288 -> [w1307]
            tunnel: w1289 -> [w1308]
            tunnel: w1290 -> [w1309]
            tunnel: w1291 -> [w1310]
            tunnel: [w1310] -> w1218
            tunnel: [w1309] -> w1217
            tunnel: [w1308] -> w1216
            tunnel: [w1307] -> w1215
            tunnel: [w1306] -> w1214
            tunnel: [w1305] -> w1213
            tunnel: [w1304] -> w1212
            tunnel: [w1303] -> w1211
            tunnel: [w1302] -> w1210
            tunnel: [w1301] -> w1209
            tunnel: [w1300] -> w1208
            tunnel: [w1299] -> w1207
            tunnel: w1206 -> [w1295]
            tunnel: [w1294] -> w1204
            tunnel: w1173 -> [w1293]
            tunnel: [w1293] -> w1172
            tunnel: [w1292] -> w1170
            tunnel: w1169 -> [w1292]
            tunnel: [w1356] -> w1285
            tunnel: [w1355] -> w1283
            tunnel: [w1354] -> w1281
            tunnel: [w1353] -> w1279
            tunnel: [w1348] -> w1267
            tunnel: [w1347] -> w1264
            tunnel: [w1346] -> w1261
            tunnel: [w1345] -> w1257
            tunnel: [w1332] -> w1248
            tunnel: [w1334] -> w1244
            tunnel: [w1331] -> w1228
            tunnel: [w1330] -> w1224
            tunnel: w1218 -> [w1333]
            tunnel: w1217 -> [w1335]
            tunnel: w1216 -> [w1360]
            tunnel: w1215 -> [w1359]
            tunnel: w1214 -> [w1358]
            tunnel: w1213 -> [w1357]
            tunnel: w1212 -> [w1356]
            tunnel: w1211 -> [w1355]
            tunnel: w1210 -> [w1354]
            tunnel: w1209 -> [w1353]
            tunnel: w1208 -> [w1346]
            tunnel: w1207 -> [w1345]
            tunnel: [w1328] -> w1205
            tunnel: w1204 -> [w1328]
            tunnel: w1172 -> [w1326]
            tunnel: w1170 -> [w1323]
            tunnel: w1285 -> [w1416]
            tunnel: w1283 -> [w1415]
            tunnel: w1281 -> [w1412]
            tunnel: w1279 -> [w1411]
            tunnel: [w1414] -> w1276
            tunnel: [w1413] -> w1275
            tunnel: [w1412] -> w1272
            tunnel: [w1411] -> w1270
            tunnel: [w1409] -> w1268
            tunnel: w1267 -> [w1409]
            tunnel: [w1408] -> w1265
            tunnel: w1264 -> [w1408]
            tunnel: [w1407] -> w1262
            tunnel: w1261 -> [w1407]
            tunnel: [w1406] -> w1258
            tunnel: w1257 -> [w1406]
            tunnel: [w1405] -> w1249
            tunnel: w1248 -> [w1405]
            tunnel: [w1404] -> w1245
            tunnel: w1244 -> [w1404]
            tunnel: [w1403] -> w1229
            tunnel: w1228 -> [w1403]
            tunnel: [w1402] -> w1225
            tunnel: w1224 -> [w1402]
            tunnel: w1205 -> [w1401]
            tunnel: [w1401] -> w1201
            tunnel: [w1430] -> w1277
            tunnel: w1276 -> [w1430]
            tunnel: w1275 -> [w1429]
            tunnel: [w1429] -> w1274
            tunnel: [w1428] -> w1273
            tunnel: w1272 -> [w1428]
            tunnel: [w1427] -> w1271
            tunnel: w1270 -> [w1427]
            tunnel: [w1426] -> w1269
            tunnel: w1268 -> [w1426]
            tunnel: [w1425] -> w1266
            tunnel: w1265 -> [w1425]
            tunnel: [w1424] -> w1263
            tunnel: w1262 -> [w1424]
            tunnel: [w1423] -> w1259
            tunnel: w1258 -> [w1423]
            tunnel: [w1422] -> w1250
            tunnel: w1249 -> [w1422]
            tunnel: [w1421] -> w1246
            tunnel: w1245 -> [w1421]
            tunnel: [w1420] -> w1230
            tunnel: w1229 -> [w1420]
            tunnel: [w1419] -> w1226
            tunnel: w1225 -> [w1419]
            tunnel: [w1418] -> w1202
            tunnel: w1201 -> [w1418]
            tunnel: w1277 -> [w1446]
            tunnel: w1274 -> [w1445]
            tunnel: [w1444] -> w1199
            tunnel: w1273 -> [w1444]
            tunnel: [w1443] -> w1197
            tunnel: w1271 -> [w1443]
            tunnel: [w1442] -> w1195
            tunnel: [w1441] -> w1193
            tunnel: [w1439] -> w1191
            tunnel: w1269 -> [w1439]
            tunnel: [w1438] -> w1189
            tunnel: w1266 -> [w1438]
            tunnel: [w1437] -> w1187
            tunnel: w1263 -> [w1437]
            tunnel: [w1436] -> w1185
            tunnel: w1259 -> [w1436]
            tunnel: [w1435] -> w1183
            tunnel: w1250 -> [w1435]
            tunnel: [w1434] -> w1181
            tunnel: w1246 -> [w1434]
            tunnel: [w1433] -> w1179
            tunnel: w1230 -> [w1433]
            tunnel: [w1432] -> w1177
            tunnel: w1226 -> [w1432]
            tunnel: [w1431] -> w1175
            tunnel: w1202 -> [w1431]
            tunnel: w1199 -> [w1463]
            tunnel: [w1463] -> w1198
            tunnel: w1197 -> [w1462]
            tunnel: [w1462] -> w1196
            tunnel: w1195 -> [w1461]
            tunnel: [w1461] -> w1194
            tunnel: w1193 -> [w1460]
            tunnel: [w1460] -> w1192
            tunnel: w1191 -> [w1452]
            tunnel: [w1451] -> w1190
            tunnel: w1189 -> [w1450]
            tunnel: [w1449] -> w1188
            tunnel: w1187 -> [w1459]
            tunnel: [w1459] -> w1186
            tunnel: w1185 -> [w1458]
            tunnel: [w1458] -> w1184
            tunnel: w1183 -> [w1457]
            tunnel: [w1457] -> w1182
            tunnel: w1181 -> [w1456]
            tunnel: [w1456] -> w1180
            tunnel: w1179 -> [w1455]
            tunnel: [w1455] -> w1178
            tunnel: w1177 -> [w1454]
            tunnel: [w1454] -> w1176
            tunnel: w1175 -> [w1453]
            tunnel: [w1453] -> w1174
            tunnel: w1198 -> [w1483]
            tunnel: w1196 -> [w1482]
            tunnel: w1194 -> [w1481]
            tunnel: w1192 -> [w1480]
            tunnel: w1190 -> [w1479]
            tunnel: w1188 -> [w1478]
            tunnel: w1186 -> [w1477]
            tunnel: w1184 -> [w1476]
            tunnel: [w1479] -> w1255
            tunnel: [w1478] -> w1254
            tunnel: [w1477] -> w1253
            tunnel: [w1476] -> w1252
            tunnel: [w1475] -> w1251
            tunnel: w1182 -> [w1475]
            tunnel: [w1474] -> w1247
            tunnel: w1180 -> [w1474]
            tunnel: [w1473] -> w1239
            tunnel: [w1472] -> w1238
            tunnel: [w1471] -> w1237
            tunnel: [w1470] -> w1236
            tunnel: [w1469] -> w1231
            tunnel: w1178 -> [w1469]
            tunnel: [w1468] -> w1227
            tunnel: w1176 -> [w1468]
            tunnel: w1219 -> [w1467]
            tunnel: [w1465] -> w1203
            tunnel: w1174 -> [w1465]
            tunnel: w1171 -> [w1464]
            tunnel: w1255 -> [w1504]
            tunnel: w1254 -> [w1503]
            tunnel: w1253 -> [w1517]
            tunnel: w1252 -> [w1516]
            tunnel: w1251 -> [w1515]
            tunnel: w1247 -> [w1514]
            tunnel: [w1515] -> w1220
            tunnel: [w1514] -> w1221
            tunnel: [w1513] -> w1243
            tunnel: [w1512] -> w1242
            tunnel: [w1504] -> w1241
            tunnel: [w1503] -> w1240
            tunnel: [w1511] -> w1232
            tunnel: w1239 -> [w1511]
            tunnel: [w1510] -> w1233
            tunnel: w1238 -> [w1510]
            tunnel: [w1509] -> w1234
            tunnel: w1237 -> [w1509]
            tunnel: [w1508] -> w1235
            tunnel: w1236 -> [w1508]
            tunnel: [w1507] -> w1222
            tunnel: w1231 -> [w1507]
            tunnel: w1227 -> [w1506]
            tunnel: [w1506] -> w1223
            tunnel: [w1505] -> w1200
            tunnel: w1203 -> [w1505]
            frame #0 {
              n353 = local read "Sweep Pattern"() -> (w1296:u8)
              n354 = local read "Current RO"() -> (w1298:u8)
              n355 = Not Equal?(x=w1296, y=w1298) -> (x != y?=w1297:bool)
              n356 = case shown="True" w1297 {
                tunnel: w1296 -> [_ w1316]
                tunnel: w1295 -> [w1311 w1314]
                tunnel: [w1311 w1312] -> w1294
                frame False {
                }
                frame True {
                  n357 = call <userlib>:"set Selected RO.vi"("error in (no error)"=w1314, "runningOrder"=w1316) -> ("error out"=w1313:errorcluster, "function return"=w1315:i16)  [unwired: 8 in]
                  n358 = case shown="0, Default" w1315 {
                    tunnel: w1313 -> [w1319 w1322]
                    tunnel: [w1317 w1322] -> w1312
                    frame 0, Default {
                      n359 = call <userlib>:"get Activation State.vi"("error in (no error)"=w1319) -> ("error out"=w1318:errorcluster, "String"=w1320:string)  [unwired: 7 in, 2 out]
                      n360 = local write "SLM State"(w1320) -> ()
                      n361 = call <userlib>:"get Selected RO.vi"("error in (no error)"=w1318) -> ("error out"=w1317:errorcluster, "selectedRO"=w1321:u8)  [unwired: 8 in, 1 out]
                      n362 = local write "Current RO"(w1321) -> ()
                    }
                    frame 1 {
                    }
                  }
                }
              }
            }
            frame #1 {
              # "Set the current voltage step"
              n363 = local read "Channel"() -> (w1329:T5)
              n364 = local read "Step index:"() -> (w1349:i16)
              n365 = local read "Max V"() -> (w1343:dbl)
              n366 = local read "Min V"() -> (w1337:dbl)
              n367 = local read "V. steps"() -> (w1342:i16)
              n368 = Quotient & Remainder(x=w1326, y=w1323) -> (x-y*floor(x/y)=w1352:i32)  [unwired: 1 out]
              n369 = To Unsigned Byte Integer(number=w1329) -> (unsigned 8bit integer=w1327:u8)
              n370 = Subtract(x=w1343, y=w1337) -> (x-y=w1341:dbl)
              n371 = Decrement(x=w1342) -> (x-1=w1340:i16)
              n372 = Equal?(x=w1352, y=0) -> (x = y?=w1344:bool)
              n373 = Divide(x=w1341, y=w1340) -> (x/y=w1339:dbl)
              n374 = case shown="2" w1327 {
                tunnel: w1360 -> [w1378 w1384 w1400]
                tunnel: w1359 -> [w1377 w1383 w1399]
                tunnel: [w1376 w1386 w1398] -> w1348
                tunnel: [w1375 w1385 w1397] -> w1347
                tunnel: w1357 -> [w1374 w1389 w1396]
                tunnel: [w1372 w1387 w1395] -> w1331
                tunnel: w1358 -> [w1371 w1382 w1393]
                tunnel: [w1370 w1381 w1392] -> w1330
                frame 0, Default {
                  w1368 = bool[] [TRUE, FALSE, FALSE] ("data")
                  # "Wavelength 0: 488nm"
                  n375 = VISA Write(VISA resource name=w1371, write buffer="7 1,4\r", error in (no error)=w1374) -> (VISA resource name out=w1372:refnum<visa-resource-name>, error out=w1370:errorcluster)  [unwired: 1 out]
                  n376 = call-poly <vilib>:"DAQmx Write.vi"("task/channels in"=w1378, "data"=w1368, "error in"=w1377) -> ("task out"=w1376:refnum<k21>, "error out"=w1375:errorcluster)  [unwired: 10 in, 1 out]
                  n377 = Array To Cluster(array=w1368) -> (cluster=w1369:T12)
                  n378 = local write "Laser Cluster"(w1369) -> ()
                }
                frame 1 {
                  w1380 = bool[] [FALSE, FALSE, TRUE] ("data")
                  # "Wavelength 2: 561 nm"
                  n379 = Array To Cluster(array=w1380) -> (cluster=w1379:T12)
                  n380 = local write "Laser Cluster"(w1379) -> ()
                  n381 = VISA Write(VISA resource name=w1382, write buffer="7 1,3\r", error in (no error)=w1389) -> (VISA resource name out=w1387:refnum<visa-resource-name>, error out=w1381:errorcluster)  [unwired: 1 out]
                  n382 = call-poly <vilib>:"DAQmx Write.vi"("task/channels in"=w1384, "data"=w1380, "error in"=w1383) -> ("task out"=w1386:refnum<k21>, "error out"=w1385:errorcluster)  [unwired: 10 in, 1 out]
                }
                frame 2 {
                  w1390 = bool[] [FALSE, TRUE, FALSE] ("data")
                  # "Wavelength 1: 640nm"
                  n383 = Array To Cluster(array=w1390) -> (cluster=w1391:T12)
                  n384 = local write "Laser Cluster"(w1391) -> ()
                  n385 = call-poly <vilib>:"DAQmx Write.vi"("task/channels in"=w1400, "data"=w1390, "error in"=w1399) -> ("task out"=w1398:refnum<k21>, "error out"=w1397:errorcluster)  [unwired: 10 in, 1 out]
                  n386 = VISA Write(VISA resource name=w1393, write buffer="7 1,2\r", error in (no error)=w1396) -> (VISA resource name out=w1395:refnum<visa-resource-name>, error out=w1392:errorcluster)  [unwired: 1 out]
                }
              }
              n387 = Increment(x=w1349) -> (x+1=w1350:i16)
              n388 = Select(t=w1350, s=w1344, f=w1349) -> (s? t:f=w1324:i16)
              n389 = local write "Step index:"(w1324) -> ()
              n390 = Decrement(x=w1324) -> (x-1=w1325:i16)
              n391 = Multiply(x=w1325, y=w1339) -> (x*y=w1338:dbl)
              n392 = Add(x=w1338, y=w1337) -> (x+y=w1336:dbl)
              n393 = case shown="True" w1344 {
                tunnel: w1336 -> [_ w1367]
                tunnel: w1335 -> [w1361 w1366]
                tunnel: [w1361 w1365] -> w1334
                tunnel: w1333 -> [w1362 w1364]
                tunnel: [w1362 w1363] -> w1332
                frame False {
                }
                frame True {
                  n394 = call-poly <vilib>:"DAQmx Write.vi"("task/channels in"=w1364, "data"=w1367, "error in"=w1366) -> ("task out"=w1363:refnum<k21>, "error out"=w1365:errorcluster)  [unwired: 10 in, 1 out]
                }
              }
              n395 = local write "Output Voltage"(w1336) -> ()
            }
            frame #2 {
              n396 = call-poly <vilib>:"DAQmx Write.vi"("task/channels in"=w1416, "data"=TRUE ("auto start"), "error in"=w1415) -> ("task out"=w1414:refnum<k21>, "error out"=w1413:errorcluster)  [unwired: 10 in, 1 out]
            }
            frame #3 {
              n397 = local read "Exposure\n(ms)"() -> (w1417:u32)
              n398 = Wait (ms)(milliseconds to wait=w1417) -> ()  [unwired: 1 out]
            }
            frame #4 {
              n399 = call-poly <vilib>:"DAQmx Write.vi"("task/channels in"=w1446, "data"=FALSE ("auto start"), "error in"=w1445) -> ("task out"=w1442:refnum<k21>, "error out"=w1441:errorcluster)  [unwired: 10 in, 1 out]
            }
            frame #5 {
              w1447 = bool[] [FALSE, FALSE, FALSE] ("data")
              # "Switch lasers off"
              n400 = Array To Cluster(array=w1447) -> (cluster=w1448:T12)
              n401 = local write "Laser Cluster"(w1448) -> ()
              n402 = call-poly <vilib>:"DAQmx Write.vi"("task/channels in"=w1452, "data"=w1447, "error in"=w1450) -> ("task out"=w1451:refnum<k21>, "error out"=w1449:errorcluster)  [unwired: 10 in, 1 out]
            }
            frame #6 {
              n403 = Equal?(x=w1464, y=w1467) -> (x = y?=w1466:bool)
              n404 = case shown="True" w1466 {
                tunnel: w1483 -> [w1491 w1499]
                tunnel: w1482 -> [w1490 w1500]
                tunnel: w1481 -> [w1489 w1502]
                tunnel: w1480 -> [w1488 w1501]
                tunnel: [w1487 w1502] -> w1473
                tunnel: [w1486 w1501] -> w1472
                tunnel: [w1485 w1499] -> w1471
                tunnel: [w1484 w1500] -> w1470
                frame False {
                  n405 = while {
                    tunnel: [w1498] -> w1487
                    tunnel: w1489 -> [w1498]
                    tunnel: [w1497] -> w1486
                    tunnel: w1488 -> [w1497]
                    tunnel: w1491 -> [w1496]
                    tunnel: w1490 -> [w1495]
                    tunnel: [w1494] -> w1484
                    tunnel: [w1493] -> w1485
                    stop <- w1492 stop-if-true
                    # "Wait until Trigger Ready received"
                    n406 = call-poly <vilib>:"DAQmx Read.vi"("task/channels in"=w1496, "error in"=w1495) -> ("task out"=w1493:refnum<k21>, "data"=w1492:bool, "error out"=w1494:errorcluster)  [unwired: 11 in]
                  }
                }
                frame True {
                }
              }
            }
            frame #7 {
              # "mjf: Not sure what this is for."
              n407 = call-poly <vilib>:"DAQmx Write.vi"("task/channels in"=w1517, "data"=TRUE, "error in"=w1516) -> ("task out"=w1518:refnum<k21>, "error out"=w1520:errorcluster)  [unwired: 10 in, 1 out]
              n408 = flat-sequence {
                tunnel: [w1526] -> w1521
                tunnel: w1520 -> [w1526]
                tunnel: [w1525] -> w1519
                tunnel: w1518 -> [w1525]
                frame #0 {
                  n409 = Wait (ms)(milliseconds to wait=u32 5) -> ()  [unwired: 1 out]
                }
              }
              n410 = call-poly <vilib>:"DAQmx Write.vi"("task/channels in"=w1519, "data"=TRUE, "error in"=w1521) -> ("task out"=w1513:refnum<k21>, "error out"=w1512:errorcluster)  [unwired: 10 in, 1 out]
            }
          }
          n411 = Increment(x=w1173) -> (x+1=w1219:i32)
          n412 = local write "Current \nFrame"(w1219) -> ()
        }
        n413 = flat-sequence {
          tunnel: w1123 -> [w1156]
          tunnel: w1122 -> [w1154]
          tunnel: [w1155] -> w1121
          tunnel: [w1153] -> w1120
          tunnel: [w1164] -> w1112
          tunnel: w1119 -> [w1164]
          tunnel: w1118 -> [w1163]
          tunnel: [w1163] -> w1113
          tunnel: [w1162] -> w1097
          tunnel: w1117 -> [w1162]
          tunnel: w1116 -> [w1161]
          tunnel: [w1161] -> w1096
          tunnel: w1103 -> [w1160]
          tunnel: w1115 -> [w1159]
          tunnel: [w1160] -> w1114
          tunnel: [w1159] -> w1100
          tunnel: [w1158] -> w1110
          tunnel: w1111 -> [w1158]
          tunnel: w1108 -> [w1157]
          tunnel: [w1157] -> w1109
          tunnel: w1102 -> [w1151]
          tunnel: [w1151] -> w1101
          tunnel: [w1150] -> w1098
          tunnel: w1099 -> [w1150]
          frame #0 {
            n414 = call-poly <vilib>:"DAQmx Write.vi"("task/channels in"=w1156, "data"=0.0, "error in"=w1154) -> ("task out"=w1155:refnum<k21>, "error out"=w1153:errorcluster)  [unwired: 10 in, 1 out]
            n415 = local write "Sweep"(FALSE ("LCVR sweep")) -> ()
          }
        }
      }
      event "Sweep Pattern", "V. steps": Value Change {
        n416 = event-data() -> ()  [unwired: 1 in, 1 out]
        n417 = local read "Sweep Pattern"() -> (w1543:u8)
        n418 = case shown="21..23, Default" w1543 {
          tunnel: [9 12 15] -> w1544
          frame 21..23, Default {
          }
          frame 24..26 {
          }
          frame 27..29 {
          }
        }
        n419 = local read "V. steps"() -> (w1545:i16)
        n420 = Multiply(x=w1545, y=w1544) -> (x*y=w1546:i32)
        n421 = local write "Total Sweep Images:"(w1546) -> ()
      }
      event "Live on": Value Change {
        n422 = event-data() -> ("NewVal"=w1564:bool)  [unwired: 1 in, 2 out]
        n423 = Select(t=2.0, s=w1564, f=0.0) -> (s? t:f=w1551:dbl)
        n424 = property on="Add bkmk" class="Bool (strict)"("DisabledEnum"=w1551) -> ()  [unwired: 2 in, 2 out]
        n425 = property on="Delete bkmk" class="Bool (strict)"("DisabledEnum"=w1551) -> ()  [unwired: 2 in, 2 out]
        n426 = property on="Clear table" class="Bool (strict)"("DisabledEnum"=w1551) -> ()  [unwired: 2 in, 2 out]
        n427 = property on="Exp 2" class="DigNum (strict)"("DisabledEnum"=w1551) -> ()  [unwired: 2 in, 2 out]
        n428 = property on="Exp 1" class="DigNum (strict)"("DisabledEnum"=w1551) -> ()  [unwired: 2 in, 2 out]
        n429 = property on="Acquire" class="Bool (strict)"("DisabledEnum"=w1551) -> ()  [unwired: 2 in, 2 out]
        n430 = property on="#t-frames" class="DigNum (strict)"("DisabledEnum"=w1551) -> ()  [unwired: 2 in, 2 out]
        n431 = property on="t-interval" class="DigNum (strict)"("DisabledEnum"=w1551) -> ()  [unwired: 2 in, 2 out]
        n432 = property on="Int unit" class="Enum (strict)"("DisabledEnum"=w1551) -> ()  [unwired: 2 in, 2 out]
        n433 = property on="Exp 0" class="DigNum (strict)"("DisabledEnum"=w1551) -> ()  [unwired: 2 in, 2 out]
        n434 = property on="Create grid" class="Bool (strict)"("DisabledEnum"=w1551) -> ()  [unwired: 2 in, 2 out]
        n435 = property on="z-step (um)" class="DigNum (strict)"("DisabledEnum"=w1551) -> ()  [unwired: 2 in, 2 out]
        n436 = property on="#z-planes" class="DigNum (strict)"("DisabledEnum"=w1551) -> ()  [unwired: 2 in, 2 out]
        n437 = property on="#Channels" class="DigNum (strict)"("DisabledEnum"=w1551) -> ()  [unwired: 2 in, 2 out]
        n438 = property on="Optosplit" class="Bool (strict)"("DisabledEnum"=w1551) -> ()  [unwired: 2 in, 2 out]
        n439 = property on="Tab Control" class="TabCtl (strict)"("DisabledEnum"=w1551) -> ()  [unwired: 2 in, 2 out]
        n440 = case shown="True" w1564 {
          tunnel: w1584 -> [w1597 w1633]
          tunnel: w1583 -> [w1593 w1632]
          tunnel: w1582 -> [w1592 w1631]
          tunnel: w1581 -> [w1596 w1630]
          tunnel: w1580 -> [w1599 w1629]
          tunnel: w1579 -> [w1598 w1628]
          tunnel: w1578 -> [w1603 w1627]
          tunnel: w1577 -> [w1602 w1626]
          tunnel: w1576 -> [w1601 w1625]
          tunnel: w1575 -> [w1600 w1624]
          tunnel: [w1595 w1623] -> w1568
          tunnel: [w1603 w1622] -> w1574
          tunnel: [w1602 w1621] -> w1573
          tunnel: [w1601 w1620] -> w1572
          tunnel: [w1600 w1619] -> w1571
          tunnel: [w1599 w1618] -> w1570
          tunnel: [w1598 w1617] -> w1569
          tunnel: [w1594 w1614] -> w1567
          tunnel: [w1593 w1616] -> w1565
          tunnel: [w1592 w1615] -> w1566
          tunnel: [w1591 w1613] -> w1561
          tunnel: w1560 -> [w1591 w1612]
          tunnel: w1559 -> [w1590 w1611]
          tunnel: [w1590 w1610] -> w1558
          tunnel: w1557 -> [w1589 w1609]
          tunnel: [w1589 w1608] -> w1556
          tunnel: w1555 -> [w1588 w1607]
          tunnel: w1554 -> [w1587 w1606]
          tunnel: [w1587 w1604] -> w1552
          tunnel: [w1588 w1605] -> w1553
          frame False {
            w1585 = bool[] [FALSE, FALSE, FALSE] ("data")
            # "Turn off all lasers"
            n441 = call-poly <vilib>:"DAQmx Write.vi"("task/channels in"=w1597, "data"=w1585, "error in"=w1596) -> ("task out"=w1595:refnum<k21>, "error out"=w1594:errorcluster)  [unwired: 10 in, 1 out]
            n442 = Array To Cluster(array=w1585) -> (cluster=w1586:T12)
            n443 = local write "Laser Cluster"(w1586) -> ()
          }
          frame True {
            n444 = while {
              tunnel: w1633 -> [w1776]
              tunnel: w1632 -> [w1775]
              tunnel: w1631 -> [w1774]
              tunnel: w1630 -> [w1773]
              tunnel: w1629 -> [w1772]
              tunnel: w1628 -> [w1771]
              tunnel: w1627 -> [w1769]
              tunnel: w1626 -> [w1767]
              tunnel: w1625 -> [w1759]
              tunnel: w1624 -> [w1755]
              tunnel: [w1751] -> w1623
              tunnel: [w1749] -> w1622
              tunnel: [w1748] -> w1621
              tunnel: [w1747] -> w1620
              tunnel: [w1746] -> w1619
              tunnel: [w1742] -> w1618
              tunnel: [w1738] -> w1617
              tunnel: [w1734] -> w1616
              tunnel: [w1730] -> w1615
              tunnel: [w1726] -> w1614
              tunnel: [w1674] -> w1613
              tunnel: w1612 -> [w1702]
              tunnel: w1611 -> [w1673]
              tunnel: [w1665] -> w1610
              tunnel: w1609 -> [w1664]
              tunnel: [w1656] -> w1608
              tunnel: w1607 -> [w1654]
              tunnel: w1606 -> [w1655]
              tunnel: [w1651] -> w1605
              tunnel: [w1644] -> w1604
              stop <- w1750 stop-if-true
              n445 = flat-sequence {
                tunnel: w1755 -> [w1797]
                tunnel: w1759 -> [w1798]
                tunnel: w1767 -> [w1799]
                tunnel: w1769 -> [w1800]
                tunnel: w1771 -> [w1801]
                tunnel: w1772 -> [w1802]
                tunnel: w1773 -> [w1803]
                tunnel: w1774 -> [w1804]
                tunnel: w1775 -> [w1805]
                tunnel: w1776 -> [w1806]
                tunnel: [w1806] -> w1712
                tunnel: [w1805] -> w1711
                tunnel: [w1804] -> w1710
                tunnel: [w1803] -> w1709
                tunnel: [w1802] -> w1708
                tunnel: [w1801] -> w1707
                tunnel: [w1800] -> w1706
                tunnel: [w1799] -> w1705
                tunnel: [w1798] -> w1704
                tunnel: [w1797] -> w1703
                tunnel: w1702 -> [w1794]
                tunnel: [w1793] -> w1675
                tunnel: w1673 -> [w1792]
                tunnel: [w1792] -> w1670
                tunnel: w1664 -> [w1791]
                tunnel: [w1791] -> w1662
                tunnel: w1655 -> [w1790]
                tunnel: w1654 -> [w1789]
                tunnel: [w1788] -> w1653
                tunnel: [w1787] -> w1652
                tunnel: [w1777] -> w1634
                tunnel: [w1860] -> w1770
                tunnel: [w1859] -> w1768
                tunnel: [w1858] -> w1762
                tunnel: [w1857] -> w1758
                tunnel: [w1845] -> w1752
                tunnel: [w1856] -> w1743
                tunnel: [w1855] -> w1739
                tunnel: [w1842] -> w1735
                tunnel: [w1843] -> w1731
                tunnel: [w1844] -> w1727
                tunnel: w1712 -> [w1846]
                tunnel: w1711 -> [w1848]
                tunnel: w1710 -> [w1849]
                tunnel: w1709 -> [w1847]
                tunnel: w1708 -> [w1862]
                tunnel: w1707 -> [w1861]
                tunnel: w1706 -> [w1860]
                tunnel: w1705 -> [w1859]
                tunnel: w1704 -> [w1858]
                tunnel: w1703 -> [w1857]
                tunnel: [w1854] -> w1676
                tunnel: w1675 -> [w1854]
                tunnel: [w1853] -> w1671
                tunnel: w1670 -> [w1853]
                tunnel: [w1852] -> w1663
                tunnel: w1662 -> [w1852]
                tunnel: w1653 -> [w1851]
                tunnel: w1652 -> [w1850]
                tunnel: [w1851] -> w1650
                tunnel: [w1850] -> w1638
                tunnel: w1634 -> [w1841]
                tunnel: w1770 -> [w1970]
                tunnel: w1768 -> [w1969]
                tunnel: [w1968] -> w1765
                tunnel: [w1967] -> w1764
                tunnel: w1762 -> [w1966]
                tunnel: [w1966] -> w1761
                tunnel: w1758 -> [w1965]
                tunnel: [w1965] -> w1757
                tunnel: [w1964] -> w1753
                tunnel: w1752 -> [w1964]
                tunnel: [w1963] -> w1744
                tunnel: w1743 -> [w1963]
                tunnel: [w1962] -> w1740
                tunnel: w1739 -> [w1962]
                tunnel: [w1961] -> w1736
                tunnel: w1735 -> [w1961]
                tunnel: [w1960] -> w1732
                tunnel: w1731 -> [w1960]
                tunnel: [w1959] -> w1728
                tunnel: w1727 -> [w1959]
                tunnel: [w1958] -> w1677
                tunnel: w1676 -> [w1958]
                tunnel: [w1957] -> w1672
                tunnel: w1671 -> [w1957]
                tunnel: w1663 -> [w1956]
                tunnel: [w1956] -> w1657
                tunnel: w1650 -> [w1955]
                tunnel: [w1955] -> w1649
                tunnel: [w1954] -> w1640
                tunnel: w1638 -> [w1954]
                tunnel: [w1989] -> w1766
                tunnel: w1765 -> [w1989]
                tunnel: w1764 -> [w1988]
                tunnel: [w1988] -> w1763
                tunnel: w1761 -> [w1987]
                tunnel: [w1987] -> w1760
                tunnel: w1757 -> [w1986]
                tunnel: [w1986] -> w1756
                tunnel: [w1985] -> w1754
                tunnel: w1753 -> [w1985]
                tunnel: [w1984] -> w1745
                tunnel: w1744 -> [w1984]
                tunnel: [w1983] -> w1741
                tunnel: w1740 -> [w1983]
                tunnel: [w1982] -> w1737
                tunnel: w1736 -> [w1982]
                tunnel: [w1981] -> w1733
                tunnel: w1732 -> [w1981]
                tunnel: [w1980] -> w1729
                tunnel: w1728 -> [w1980]
                tunnel: [w1979] -> w1678
                tunnel: w1677 -> [w1979]
                tunnel: w1672 -> [w1978]
                tunnel: [w1978] -> w1666
                tunnel: [w1977] -> w1658
                tunnel: w1657 -> [w1977]
                tunnel: w1649 -> [w1976]
                tunnel: [w1976] -> w1648
                tunnel: w1640 -> [w1975]
                tunnel: [w1975] -> w1639
                tunnel: ["Bleach-\nsave ratio"] -> w1635
                tunnel: w1766 -> [w2007]
                tunnel: w1763 -> [w2006]
                tunnel: w1760 -> [w2005]
                tunnel: [w2005] -> w1701
                tunnel: w1756 -> [w2004]
                tunnel: [w2004] -> w1699
                tunnel: [w2003] -> w1697
                tunnel: w1754 -> [w2003]
                tunnel: [w2002] -> w1695
                tunnel: [w2001] -> w1693
                tunnel: [w2000] -> w1691
                tunnel: w1745 -> [w2000]
                tunnel: [w1999] -> w1689
                tunnel: w1741 -> [w1999]
                tunnel: [w1998] -> w1687
                tunnel: w1737 -> [w1998]
                tunnel: [w1997] -> w1685
                tunnel: w1733 -> [w1997]
                tunnel: [w1996] -> w1683
                tunnel: w1729 -> [w1996]
                tunnel: [w1995] -> w1679
                tunnel: w1678 -> [w1995]
                tunnel: [w1994] -> w1667
                tunnel: w1666 -> [w1994]
                tunnel: [w1993] -> w1659
                tunnel: w1658 -> [w1993]
                tunnel: w1648 -> [w1992]
                tunnel: [w1992] -> w1647
                tunnel: [w1991] -> w1641
                tunnel: w1639 -> [w1991]
                tunnel: [w1990] -> w1636
                tunnel: w1635 -> [w1990]
                tunnel: w1701 -> [w2028]
                tunnel: [w2028] -> w1700
                tunnel: w1699 -> [w2027]
                tunnel: [w2027] -> w1698
                tunnel: w1697 -> [w2018]
                tunnel: [w2017] -> w1696
                tunnel: w1695 -> [w2026]
                tunnel: [w2026] -> w1694
                tunnel: w1693 -> [w2025]
                tunnel: [w2025] -> w1692
                tunnel: w1691 -> [w2024]
                tunnel: [w2024] -> w1690
                tunnel: w1689 -> [w2023]
                tunnel: [w2023] -> w1688
                tunnel: w1687 -> [w2022]
                tunnel: [w2022] -> w1686
                tunnel: w1685 -> [w2021]
                tunnel: [w2021] -> w1684
                tunnel: w1683 -> [w2020]
                tunnel: [w2019] -> w1682
                tunnel: [w2016] -> w1680
                tunnel: w1679 -> [w2016]
                tunnel: [w2015] -> w1668
                tunnel: w1667 -> [w2015]
                tunnel: [w2014] -> w1660
                tunnel: w1659 -> [w2014]
                tunnel: w1647 -> [w2013]
                tunnel: [w2013] -> w1646
                tunnel: [w2012] -> w1642
                tunnel: w1641 -> [w2012]
                tunnel: [w2011] -> w1637
                tunnel: w1636 -> [w2011]
                tunnel: w1700 -> [w2050]
                tunnel: w1698 -> [w2049]
                tunnel: w1696 -> [w2048]
                tunnel: w1694 -> [w2047]
                tunnel: w1692 -> [w2046]
                tunnel: w1690 -> [w2043]
                tunnel: w1688 -> [w2042]
                tunnel: w1686 -> [w2041]
                tunnel: w1684 -> [w2040]
                tunnel: w1682 -> [w2039]
                tunnel: [w2048] -> w1722
                tunnel: [w2047] -> w1721
                tunnel: [w2046] -> w1720
                tunnel: [w2045] -> w1719
                tunnel: [w2044] -> w1718
                tunnel: [w2043] -> w1717
                tunnel: [w2042] -> w1716
                tunnel: [w2041] -> w1715
                tunnel: [w2040] -> w1714
                tunnel: [w2039] -> w1713
                tunnel: [w2038] -> w1681
                tunnel: w1680 -> [w2038]
                tunnel: [w2037] -> w1669
                tunnel: w1668 -> [w2037]
                tunnel: [w2036] -> w1661
                tunnel: w1660 -> [w2036]
                tunnel: w1646 -> [w2035]
                tunnel: [w2035] -> w1645
                tunnel: [w2034] -> w1643
                tunnel: w1642 -> [w2034]
                tunnel: w1637 -> [w2030]
                tunnel: [w2063] -> w1726
                tunnel: [w2064] -> w1730
                tunnel: [w2065] -> w1734
                tunnel: [w2066] -> w1738
                tunnel: [w2067] -> w1742
                tunnel: [w2068] -> w1746
                tunnel: [w2069] -> w1747
                tunnel: [w2070] -> w1748
                tunnel: [w2071] -> w1749
                tunnel: [w2072] -> w1751
                tunnel: w1722 -> [w2072]
                tunnel: w1721 -> [w2071]
                tunnel: w1720 -> [w2070]
                tunnel: w1719 -> [w2069]
                tunnel: w1718 -> [w2068]
                tunnel: w1717 -> [w2067]
                tunnel: w1716 -> [w2066]
                tunnel: w1715 -> [w2065]
                tunnel: w1714 -> [w2064]
                tunnel: w1713 -> [w2063]
                tunnel: [w2062] -> w1723
                tunnel: [w2061] -> w1725
                tunnel: [w2060] -> w1674
                tunnel: w1681 -> [w2060]
                tunnel: [w2059] -> w1665
                tunnel: w1669 -> [w2059]
                tunnel: [w2058] -> w1656
                tunnel: w1661 -> [w2058]
                tunnel: [w2057] -> w1651
                tunnel: w1645 -> [w2057]
                tunnel: [w2056] -> w1644
                tunnel: w1643 -> [w2056]
                frame #0 {
                  # "Change RO if requried"
                  # "Get required RO"
                  # "Set SLM pattern"
                  n446 = local read "Optosplit"() -> (w1777:bool)
                  n447 = local read "Channel"() -> (w1782:T5)
                  n448 = local read "Preview view"() -> (w1780:T4)
                  n449 = Select(t=u8 1, s=w1777, f=w1782) -> (s? t:f=w1783:u32)
                  n450 = event shown="[0] \"Bookmark List\": Double Click" {
                    selector: _ -> [_ _]
                    dyn-events: _ -> [_ _]
                    timeout: 0 -> [_ _]
                    tunnel: w1789 -> [w1811 w1828]
                    tunnel: w1790 -> [w1810 w1827]
                    tunnel: [w1809 w1827] -> w1787
                    tunnel: [w1808 w1828] -> w1788
                    event "Bookmark List": Double Click {
                      w1819 = u16 1 items=["X", "Y", "Z"] ("Axis")
                      w1826 = u16 0 items=["X", "Y", "Z"] ("Axis")
                      n451 = event-data() -> ()  [unwired: 1 in, 8 out]
                      n452 = local read "Bookmark List"() -> (w1807:i32)
                      n453 = property on="Bookmark List" class="MCListbox (strict)"() -> ("ItemNames"=w1823:string[][])  [unwired: 2 in, 2 out]
                      n454 = Index Array(array=w1823, index (row)=w1807, index (col)=1 ("disabled index (col)")) -> (element=w1822:string)
                      n455 = Index Array(array=w1823, index (row)=w1807, index (col)=2 ("disabled index (col)")) -> (element=w1817:string)
                      n456 = Decimal String To Number(string=w1817) -> (number=w1812:i32)  [unwired: 2 in, 1 out]
                      n457 = Decimal String To Number(string=w1822) -> (number=w1815:i32)  [unwired: 2 in, 1 out]
                      n458 = To Double Precision Float(number=w1815) -> (double precision float=w1814:dbl)
                      n459 = call "ASI_move_serial.vi"("Position/distance (um)"=w1814, "error in"=w1810, "Relative?"=FALSE, "Axis"=w1826, "VISA resource name"=w1811) -> ("error out"=w1816:errorcluster, "VISA resource name out"=w1820:refnum<visa-resource-name>)  [unwired: 2 in]
                      n460 = To Double Precision Float(number=w1812) -> (double precision float=w1813:dbl)
                      n461 = call "ASI_move_serial.vi"("Position/distance (um)"=w1813, "error in"=w1816, "Relative?"=FALSE, "Axis"=w1819, "VISA resource name"=w1820) -> ("error out"=w1809:errorcluster, "VISA resource name out"=w1808:refnum<visa-resource-name>)  [unwired: 2 in]
                    }
                    event Timeout {
                      n462 = event-data() -> ()  [unwired: 1 in, 2 out]
                    }
                  }
                  n463 = local read "Manual SLM mode"() -> (w1784:bool)
                  n464 = call "RO from WL and mode.vi"("Mode"=w1780, "Wavelength"=w1783) -> ("SLM pattern"=w1779:u8)  [unwired: 9 in]
                  n465 = local read "RO"() -> (w1785:u8)
                  n466 = local read "Current RO"() -> (w1795:u8)
                  n467 = Select(t=w1785, s=w1784, f=w1779) -> (s? t:f=w1778:u8)
                  n468 = Not Equal?(x=w1778, y=w1795) -> (x != y?=w1796:bool)
                  n469 = case shown="True" w1796 {
                    tunnel: w1778 -> [_ w1834]
                    tunnel: w1794 -> [w1829 w1832]
                    tunnel: [w1829 w1830] -> w1793
                    frame False {
                    }
                    frame True {
                      n470 = call <userlib>:"set Selected RO.vi"("error in (no error)"=w1832, "runningOrder"=w1834) -> ("error out"=w1831:errorcluster, "function return"=w1833:i16)  [unwired: 8 in]
                      n471 = case shown="0, Default" w1833 {
                        tunnel: w1831 -> [w1837 w1840]
                        tunnel: [w1835 w1840] -> w1830
                        frame 0, Default {
                          n472 = call <userlib>:"get Activation State.vi"("error in (no error)"=w1837) -> ("error out"=w1836:errorcluster, "String"=w1838:string)  [unwired: 7 in, 2 out]
                          n473 = local write "SLM State"(w1838) -> ()
                          n474 = call <userlib>:"get Selected RO.vi"("error in (no error)"=w1836) -> ("error out"=w1835:errorcluster, "selectedRO"=w1839:u8)  [unwired: 8 in, 1 out]
                          n475 = local write "Current RO"(w1839) -> ()
                        }
                        frame 1 {
                        }
                      }
                    }
                  }
                }
                frame #1 {
                  # "Set laser, filter, SLM"
                  n476 = case shown="True" w1841 {
                    tunnel: w1849 -> [w1871 w1939]
                    tunnel: w1848 -> [w1870 w1940]
                    tunnel: w1847 -> [w1869 w1945]
                    tunnel: w1846 -> [w1868 w1946]
                    tunnel: [w1867 w1943] -> w1845
                    tunnel: [w1866 w1944] -> w1844
                    tunnel: [w1865 w1938] -> w1843
                    tunnel: [w1864 w1937] -> w1842
                    frame False {
                      n477 = local read "Channel"() -> (w1873:T5)
                      n478 = To Unsigned Byte Integer(number=w1873) -> (unsigned 8bit integer=w1872:u8)
                      n479 = case shown="0, Default" w1872 {
                        tunnel: w1868 -> [w1887 w1905 w1927]
                        tunnel: w1869 -> [w1886 w1904 w1926]
                        tunnel: [w1885 w1907 w1925] -> w1867
                        tunnel: w1870 -> [w1882 w1899 w1920]
                        tunnel: w1871 -> [w1883 w1898 w1921]
                        tunnel: [w1881 w1900 w1919] -> w1864
                        tunnel: [w1880 w1901 w1918] -> w1865
                        tunnel: [w1884 w1906 w1924] -> w1866
                        frame 0, Default {
                          w1874 = bool[] [TRUE, FALSE, FALSE] ("data")
                          # "Wavelength 0: 488nm"
                          n480 = local read "Current filter"() -> (w1878:string)
                          n481 = local read "Filter 488"() -> (w1877:i8)
                          n482 = Number To Decimal String(number=w1877) -> (decimal integer string=w1876:string)  [unwired: 1 in]
                          n483 = Equal?(x=w1876, y=w1878) -> (x = y?=w1879:bool)
                          n484 = case shown="False" w1879 {
                            tunnel: w1883 -> [w1891 w1892]
                            tunnel: w1882 -> [w1889 w1893]
                            tunnel: w1876 -> [w1888 _]
                            tunnel: [w1889 w1893] -> w1881
                            tunnel: [w1890 w1892] -> w1880
                            frame False {
                              n485 = call "Change_filter.vi"("error in"=w1891, "filter number"=w1888, "VISA resource name"=w1889) -> ("error out"=w1890:errorcluster)  [unwired: 7 in, 1 out]
                              n486 = local write "Current filter"(w1888) -> ()
                            }
                            frame True {
                            }
                          }
                          n487 = call-poly <vilib>:"DAQmx Write.vi"("task/channels in"=w1887, "data"=w1874, "error in"=w1886) -> ("task out"=w1885:refnum<k21>, "error out"=w1884:errorcluster)  [unwired: 10 in, 1 out]
                          n488 = Array To Cluster(array=w1874) -> (cluster=w1875:T12)
                          n489 = local write "Laser Cluster"(w1875) -> ()
                        }
                        frame 1 {
                          w1894 = bool[] [FALSE, FALSE, TRUE] ("data")
                          # "Wavelength 2: 561 nm"
                          n490 = local read "Filter 561"() -> (w1897:i8)
                          n491 = local read "Current filter"() -> (w1902:string)
                          n492 = Number To Decimal String(number=w1897) -> (decimal integer string=w1896:string)  [unwired: 1 in]
                          n493 = Equal?(x=w1896, y=w1902) -> (x = y?=w1903:bool)
                          n494 = case shown="False" w1903 {
                            tunnel: w1898 -> [w1911 w1912]
                            tunnel: w1899 -> [w1909 w1913]
                            tunnel: w1896 -> [w1908 _]
                            tunnel: [w1909 w1913] -> w1900
                            tunnel: [w1910 w1912] -> w1901
                            frame False {
                              n495 = call "Change_filter.vi"("error in"=w1911, "filter number"=w1908, "VISA resource name"=w1909) -> ("error out"=w1910:errorcluster)  [unwired: 7 in, 1 out]
                              n496 = local write "Current filter"(w1908) -> ()
                            }
                            frame True {
                            }
                          }
                          n497 = call-poly <vilib>:"DAQmx Write.vi"("task/channels in"=w1905, "data"=w1894, "error in"=w1904) -> ("task out"=w1907:refnum<k21>, "error out"=w1906:errorcluster)  [unwired: 10 in, 1 out]
                          n498 = Array To Cluster(array=w1894) -> (cluster=w1895:T12)
                          n499 = local write "Laser Cluster"(w1895) -> ()
                        }
                        frame 2 {
                          w1914 = bool[] [FALSE, TRUE, FALSE] ("data")
                          # "Wavelength 1: 640nm"
                          n500 = local read "Filter 640"() -> (w1917:i8)
                          n501 = local read "Current filter"() -> (w1922:string)
                          n502 = Number To Decimal String(number=w1917) -> (decimal integer string=w1916:string)  [unwired: 1 in]
                          n503 = Equal?(x=w1916, y=w1922) -> (x = y?=w1923:bool)
                          n504 = call-poly <vilib>:"DAQmx Write.vi"("task/channels in"=w1927, "data"=w1914, "error in"=w1926) -> ("task out"=w1925:refnum<k21>, "error out"=w1924:errorcluster)  [unwired: 10 in, 1 out]
                          n505 = case shown="False" w1923 {
                            tunnel: w1921 -> [w1931 w1932]
                            tunnel: w1920 -> [w1929 w1933]
                            tunnel: w1916 -> [w1928 _]
                            tunnel: [w1929 w1933] -> w1919
                            tunnel: [w1930 w1932] -> w1918
                            frame False {
                              n506 = call "Change_filter.vi"("error in"=w1931, "filter number"=w1928, "VISA resource name"=w1929) -> ("error out"=w1930:errorcluster)  [unwired: 7 in, 1 out]
                              n507 = local write "Current filter"(w1928) -> ()
                            }
                            frame True {
                            }
                          }
                          n508 = Array To Cluster(array=w1914) -> (cluster=w1915:T12)
                          n509 = local write "Laser Cluster"(w1915) -> ()
                        }
                      }
                    }
                    frame True {
                      n510 = local read "Filter Optosplit"() -> (w1936:i8)
                      n511 = local read "Current filter"() -> (w1941:string)
                      n512 = Cluster To Array(cluster="Live OS Channel Cluster") -> (array=w1947:bool[])
                      n513 = Number To Decimal String(number=w1936) -> (decimal integer string=w1935:string)  [unwired: 1 in]
                      n514 = Equal?(x=w1935, y=w1941) -> (x = y?=w1942:bool)
                      n515 = case shown="False" w1942 {
                        tunnel: w1939 -> [w1951 w1952]
                        tunnel: w1940 -> [w1949 w1953]
                        tunnel: w1935 -> [w1948 _]
                        tunnel: [w1949 w1953] -> w1937
                        tunnel: [w1950 w1952] -> w1938
                        frame False {
                          n516 = call "Change_filter.vi"("error in"=w1951, "filter number"=w1948, "VISA resource name"=w1949) -> ("error out"=w1950:errorcluster)  [unwired: 7 in, 1 out]
                          n517 = local write "Current filter"(w1948) -> ()
                        }
                        frame True {
                        }
                      }
                      n518 = local write "Laser Cluster"("Live OS Channel Cluster") -> ()
                      n519 = call-poly <vilib>:"DAQmx Write.vi"("task/channels in"=w1946, "data"=w1947, "error in"=w1945) -> ("task out"=w1943:refnum<k21>, "error out"=w1944:errorcluster)  [unwired: 10 in, 1 out]
                    }
                  }
                  n520 = call-poly <vilib>:"DAQmx Write.vi"("task/channels in"=w1862, "data"=TRUE, "error in"=w1861) -> ("task out"=w1856:refnum<k21>, "error out"=w1855:errorcluster)  [unwired: 10 in, 1 out]
                }
                frame #2 {
                  # "Start camera exposure"
                  n521 = call-poly <vilib>:"DAQmx Write.vi"("task/channels in"=w1970, "data"=TRUE, "error in"=w1969) -> ("task out"=w1968:refnum<k21>, "error out"=w1967:errorcluster)  [unwired: 10 in, 1 out]
                }
                frame #3 {
                  # "Expose camera"
                  n522 = local read "Exposure\n(ms)"() -> (w1973:u32)
                  n523 = Multiply(x=w1973, y="Bleach-\nsave ratio") -> (x*y=w1974:dbl)
                  n524 = Wait (ms)(milliseconds to wait=w1974) -> ()  [unwired: 1 out]
                }
                frame #4 {
                  # "End camera exposure"
                  n525 = call-poly <vilib>:"DAQmx Write.vi"("task/channels in"=w2007, "data"=FALSE, "error in"=w2006) -> ("task out"=w2002:refnum<k21>, "error out"=w2001:errorcluster)  [unwired: 10 in, 1 out]
                }
                frame #5 {
                  w2009 = bool[] [FALSE, FALSE, FALSE] ("data")
                  n526 = Array To Cluster(array=w2009) -> (cluster=w2010:T12)
                  n527 = local write "Laser Cluster"(w2010) -> ()
                  n528 = call-poly <vilib>:"DAQmx Write.vi"("task/channels in"=w2018, "data"=w2009, "error in"=w2020) -> ("task out"=w2017:refnum<k21>, "error out"=w2019:errorcluster)  [unwired: 10 in, 1 out]
                }
                frame #6 {
                  # "Or for bleach-saver time-out, if longer"
                  # "Wait until Trigger Ready received"
                  n529 = local read "Exposure\n(ms)"() -> (w2033:u32)
                  n530 = Subtract(x=1.0, y=w2030) -> (x-y=w2029:dbl)
                  n531 = while {
                    tunnel: [w2055] -> w2045
                    tunnel: w2050 -> [w2054]
                    tunnel: w2049 -> [w2053]
                    tunnel: [w2052] -> w2044
                    stop <- w2051 stop-if-true
                    n532 = call-poly <vilib>:"DAQmx Read.vi"("task/channels in"=w2054, "error in"=w2053) -> ("task out"=w2055:refnum<k21>, "data"=w2051:bool, "error out"=w2052:errorcluster)  [unwired: 11 in]
                  }
                  n533 = Multiply(x=w2033, y=w2029) -> (x*y=w2032:dbl)
                  n534 = Wait (ms)(milliseconds to wait=w2032) -> ()  [unwired: 1 out]
                }
                frame #7 {
                  # "Stop live mode?"
                  n535 = local read "stop"() -> (w2062:bool)
                  n536 = local read "Live on"() -> (w2061:bool)
                }
              }
              n537 = Not(x=w1725) -> (.not. x?=w1724:bool)
              n538 = Or(x=w1724, y=w1723) -> (x .or. y?=w1750:bool)
            }
          }
        }
      }
      event "Create grid": Value Change {
        w2085 = u16 1 items=["X", "Y", "Z"] ("Axis")
        w2086 = u16 0 items=["X", "Y", "Z"] ("Axis")
        # "Get position of X and Y axis"
        n539 = event-data() -> ()  [unwired: 1 in, 5 out]
        n540 = call "ASI_Ask_position.vi"("error in"=w2082, "Axis"=w2086, "VISA resource name"=w2080) -> ("error out"=w2084:errorcluster, "Current Z position (um)"=w2078:dbl, "VISA resource name out"=w2083:refnum<visa-resource-name>)  [unwired: 6 in]
        n541 = call "ASI_Ask_position.vi"("error in"=w2084, "Axis"=w2085, "VISA resource name"=w2083) -> ("error out"=w2081:errorcluster, "Current Z position (um)"=w2076:dbl, "VISA resource name out"=w2079:refnum<visa-resource-name>)  [unwired: 6 in]
        n542 = call "grid creator.vi"("x-start"=w2078, "y-start"=w2076) -> ("Output array"=w2074:string[][])  [unwired: 16 in, 1 out]
        n543 = local write "Create grid"(FALSE) -> ()
        n544 = Empty Array?(array=w2074) -> (empty?=w2075:bool)
        n545 = case shown="False" w2075 {
          tunnel: w2074 -> [w2100 _]
          frame False {
            n546 = property on="Bookmark List" class="MCListbox (strict)"("ItemNames"=w2100) -> ()  [unwired: 2 in, 2 out]
          }
          frame True {
          }
        }
      }
      event "RO": Value Change {
        n547 = event-data() -> ()  [unwired: 1 in, 5 out]
        n548 = local read "RO"() -> (w2118:u8)
        n549 = call <userlib>:"set Selected RO.vi"("error in (no error)"=w2119, "runningOrder"=w2118) -> ("error out"=w2116:errorcluster, "function return"=w2117:i16)  [unwired: 8 in]
        n550 = case shown="0, Default" w2117 {
          tunnel: w2116 -> [w2125 w2126]
          tunnel: [w2121 w2126] -> w2120
          frame 0, Default {
            n551 = call <userlib>:"get Activation State.vi"("error in (no error)"=w2125) -> ("error out"=w2124:errorcluster, "String"=w2123:string)  [unwired: 7 in, 2 out]
            n552 = local write "SLM State"(w2123) -> ()
            n553 = call <userlib>:"get Selected RO.vi"("error in (no error)"=w2124) -> ("error out"=w2121:errorcluster, "selectedRO"=w2122:u8)  [unwired: 8 in, 1 out]
            n554 = local write "Current RO"(w2122) -> ()
          }
          frame 1 {
          }
        }
      }
      event "Ch 1", "Ch 2", "Ch 3", "Exp 0", "Exp 1", "Exp 2", "Ch1 TIRF", "Ch2 TIRF", "Ch3 TIRF": Value Change {
        n555 = event-data() -> ()  [unwired: 1 in, 2 out]
        n556 = local read "Ch1 TIRF"() -> (w2144:bool)
        n557 = local read "Ch2 TIRF"() -> (w2145:bool)
        n558 = local read "Ch3 TIRF"() -> (w2146:bool)
        n559 = local read "Exp 0"() -> (w2150:u32)
        n560 = local read "Exp 1"() -> (w2149:u32)
        n561 = local read "Exp 2"() -> (w2148:u32)
        n562 = local read "Ch 1"() -> (w2154:T5)
        n563 = local read "Ch 2"() -> (w2153:T5)
        n564 = local read "Ch 3"() -> (w2152:T5)
        n565 = Bundle("Ch1 TIRF"=w2144, "Ch2 TIRF"=w2145, "Ch3 TIRF"=w2146) -> (w2143:T9)  [unwired: 1 in]
        n566 = Build Array(w2150, w2149, w2148) -> (w2147:u32[])
        n567 = local write "TIRF Mode N"(w2143) -> ()
        n568 = Bundle("Ch 1"=w2154, "Ch 2"=w2153, "Ch 3"=w2152) -> (w2151:T8)  [unwired: 1 in]
        n569 = local write "Exposure times N"(w2147) -> ()
        n570 = local write "Ch N"(w2151) -> ()
      }
      event "#t-frames", "SIM Frames", "#Channels", "t-interval", "Int unit", "#z-planes", "#bookmarks", "Widefield?": Value Change {
        n571 = event-data() -> ()  [unwired: 1 in, 5 out]
        n572 = flat-sequence {
          tunnel: [w2187] -> w2181
          frame #0 {
            n573 = local read "Widefield?"() -> (w2186:bool)
            n574 = Select(t=1, s=w2186, f=9) -> (s? t:f=w2183:i32)
            n575 = local write "SIM Frames"(w2183) -> ()
          }
          frame #1 {
            n576 = local read "SIM Frames"() -> (w2187:i16)
          }
        }
        n577 = local read "#bookmarks"() -> (w2159:i16)
        n578 = local read "#t-frames"() -> (w2182:i16)
        n579 = local read "#Channels"() -> (w2179:i16)
        n580 = Equal To 0?(x=w2159) -> (x = 0?=w2158:bool)
        n581 = local read "#z-planes"() -> (w2177:i16)
        n582 = Multiply(x=w2182, y=w2181) -> (x*y=w2180:i16)
        n583 = Multiply(x=w2180, y=w2179) -> (x*y=w2178:i16)
        n584 = Select(t=i16 1, s=w2158, f=w2159) -> (s? t:f=w2156:i16)
        n585 = Multiply(x=w2178, y=w2177) -> (x*y=w2160:i16)
        n586 = Multiply(x=w2160, y=w2156) -> (x*y=w2161:i16)
        n587 = local write "Total\nFrames"(w2161) -> ()
      }
      event "z0 (um)": Value Change {
        n588 = event-data() -> ()  [unwired: 1 in, 5 out]
        n589 = local read "Z-move method"() -> (w2207:u16)
        n590 = local read "z0 (um)"() -> (w2205:dbl)
        n591 = call "WriteZ.vi"("new-z (um)"=w2205, "Method"=w2207, "error in (no error)"=w2189, "ASI VISA resource name"=w2208) -> ("error out"=w2202:errorcluster, "V"=w2206:dbl, "ASI VISA resource name OUT"=w2203:refnum<visa-resource-name>)  [unwired: 5 in]
        n592 = local write "Current piezo position (V)"(w2206) -> ()
        n593 = local write "Current z-position (um)"(w2205) -> ()
      }
      event "Add bkmk": Value Change {
        n594 = event-data() -> ()  [unwired: 1 in, 5 out]
        n595 = flat-sequence {
          tunnel: w2211 -> [w2233]
          tunnel: w2213 -> [w2234]
          tunnel: [w2234] -> w2217
          tunnel: [w2233] -> w2216
          tunnel: w2217 -> [w2244]
          tunnel: w2216 -> [w2243]
          tunnel: [w2238] -> w2215
          tunnel: [w2237] -> w2214
          tunnel: [w2236] -> w2212
          tunnel: [w2235] -> w2210
          tunnel: w2215 -> [w2263]
          tunnel: w2214 -> [w2264]
          frame #0 {
            # "For performance"
            n596 = property class="VI"() -> ("Panel"=w2232:refnum<vi>)  [unwired: 2 in, 2 out]
            n597 = property class="Pnl"(reference=w2232, "DeferPanUpdts"=TRUE ("Defer Panel Updates")) -> ()  [unwired: 1 in, 2 out]
          }
          frame #1 {
            w2241 = u16 1 items=["X", "Y", "Z"] ("Axis")
            w2242 = u16 0 items=["X", "Y", "Z"] ("Axis")
            # "Get position of X and Y axis"
            n598 = call "ASI_Ask_position.vi"("error in"=w2243, "Axis"=w2242, "VISA resource name"=w2244) -> ("error out"=w2240:errorcluster, "Current Z position (um)"=w2237:dbl, "VISA resource name out"=w2239:refnum<visa-resource-name>)  [unwired: 6 in]
            n599 = call "ASI_Ask_position.vi"("error in"=w2240, "Axis"=w2241, "VISA resource name"=w2239) -> ("error out"=w2235:errorcluster, "Current Z position (um)"=w2238:dbl, "VISA resource name out"=w2236:refnum<visa-resource-name>)  [unwired: 6 in]
          }
          frame #2 {
            # "... and add to list"
            # "Name the bookmark nicely..."
            n600 = Number To Decimal String(number=w2264) -> (decimal integer string=w2261:string)  [unwired: 1 in]
            n601 = Number To Decimal String(number=w2263) -> (decimal integer string=w2262:string)  [unwired: 1 in]
            n602 = property on="Bookmark List" class="MCListbox (strict)"() -> ("ItemNames"=w2257:string[][])  [unwired: 2 in, 2 out]
            n603 = Array Size(array=w2257) -> (size(s)=w2256:i32[])
            n604 = Index Array(array=w2256, index=0) -> (element=w2246:i32)
            n605 = Decrement(x=w2246) -> (x-1=w2245:i32)
            n606 = Index Array(array=w2257, index (row)=w2245, index (col)=0 ("disabled index (col)")) -> (element=w2252:string)
            n607 = String Subset(string=w2252, offset (0)=4) -> (substring=w2250:string)  [unwired: 1 in]
            n608 = Decimal String To Number(string=w2250) -> (number=w2249:i32)  [unwired: 2 in, 1 out]
            n609 = Increment(x=w2249) -> (x+1=w2248:i32)
            n610 = Number To Decimal String(number=w2248) -> (decimal integer string=w2247:string)  [unwired: 1 in]
            n611 = Concatenate Strings("Pos-" ("element"), w2247) -> (w2253:string)
            n612 = Build Array(w2253, w2261, w2262) -> (w2260:string[])
            n613 = Insert Into Array(array=w2257, new element=w2260) -> (w2259:string[][])  [unwired: 2 in]
            n614 = property on="Bookmark List" class="MCListbox (strict)"("ItemNames"=w2259) -> ()  [unwired: 2 in, 2 out]
          }
          frame #3 {
            # "Reset button"
            # "For performance"
            n615 = property class="VI"() -> ("Panel"=w2267:refnum<vi>)  [unwired: 2 in, 2 out]
            n616 = property class="Pnl"(reference=w2267, "DeferPanUpdts"=FALSE ("Defer Panel Updates")) -> ()  [unwired: 1 in, 2 out]
            n617 = local write "Add bkmk"(FALSE) -> ()
          }
        }
      }
      event "Save bkmk table": Value Change {
        n618 = event-data() -> ()  [unwired: 1 in, 5 out]
        n619 = property on="Bookmark List" class="MCListbox (strict)"() -> ("ItemNames"=w2270:string[][])  [unwired: 2 in, 2 out]
        n620 = local write "Save bkmk table"(FALSE ("Save bkmk table")) -> ()
        n621 = call-poly <vilib>:"Write To Spreadsheet File.vi"("2D data"=w2270) -> ()  [unwired: 7 in, 1 out]
      }
      event "Load bkmk table": Value Change {
        n622 = event-data() -> ()  [unwired: 1 in, 5 out]
        n623 = call-poly <vilib>:"Read From Spreadsheet File.vi"() -> ("all rows"=w2290:string[][], "new file path (Not A Path if cancelled)"=w2289:path)  [unwired: 7 in, 3 out]
        n624 = Path Type(1:w2289) -> (0:w2288:i16)
        n625 = local write "Load bkmk table"(FALSE ("Load bkmk table")) -> ()
        n626 = case shown="0, 1" w2288 {
          tunnel: w2290 -> [_ w2306]
          frame 2, Default {
          }
          frame 0, 1 {
            n627 = property on="Bookmark List" class="MCListbox (strict)"("ItemNames"=w2306) -> ()  [unwired: 2 in, 2 out]
          }
        }
      }
      event "Delete bkmk": Value Change {
        n628 = event-data() -> ()  [unwired: 1 in, 5 out]
        n629 = flat-sequence {
          frame #0 {
            n630 = property class="VI"() -> ("Panel"=w2323:refnum<vi>)  [unwired: 2 in, 2 out]
            n631 = property class="Pnl"(reference=w2323, "DeferPanUpdts"=TRUE ("Defer Panel Updates")) -> ()  [unwired: 1 in, 2 out]
          }
          frame #1 {
            n632 = local read "Bookmark List"() -> (w2325:i32)
            n633 = property on="Bookmark List" class="MCListbox (strict)"() -> ("ItemNames"=w2328:string[][])  [unwired: 2 in, 2 out]
            n634 = Delete From Array(array=w2328, length=1, index (row)=w2325) -> (array with subset deleted=w2326:string[][])  [unwired: 1 in, 1 out]
            n635 = property on="Bookmark List" class="MCListbox (strict)"("ItemNames"=w2326) -> ()  [unwired: 2 in, 2 out]
          }
          frame #2 {
            n636 = property class="VI"() -> ("Panel"=w2330:refnum<vi>)  [unwired: 2 in, 2 out]
            n637 = property class="Pnl"(reference=w2330, "DeferPanUpdts"=FALSE ("Defer Panel Updates")) -> ()  [unwired: 1 in, 2 out]
            n638 = local write "Delete bkmk"(FALSE ("Delete bkmk")) -> ()
          }
        }
      }
      event "Clear table": Value Change {
        n639 = event-data() -> ()  [unwired: 1 in, 5 out]
        n640 = Initialize Array("string" ("format string"), 0 ("dimension size"), 3 ("dimension size")) -> (w2335:string[][])
        n641 = property on="Bookmark List" class="MCListbox (strict)"("ItemNames"=w2335) -> ()  [unwired: 2 in, 2 out]
        n642 = local write "Clear table"(FALSE ("Clear table")) -> ()
      }
      event "Open Logbook": Value Change {
        n643 = event-data() -> ("NewVal"=w2355:bool)  [unwired: 1 in, 4 out]
        n644 = case shown="True" w2355 {
          frame False {
          }
          frame True {
            n645 = call-poly <vilib>:"Open URL in Default Browser.vi"("URL"="https://www.labstep.com/app/#/timeline") -> ()  [unwired: 5 in, 2 out]
          }
        }
        n646 = local write "Open Logbook"(FALSE ("Open Logbook")) -> ()
      }
      event "Post to logbook": Value Change {
        n647 = event-data() -> ("NewVal"=w2378:bool)  [unwired: 1 in, 5 out]
        n648 = local read "Logbook entry"() -> (w2377:string)
        n649 = String Length(string=w2377) -> (length=w2374:i32)
        n650 = Less?(x=1, y=w2374) -> (x < y?=w2373:bool)
        n651 = And(x=w2378, y=w2373) -> (x .and. y?=w2379:bool)
        n652 = case shown="True" w2379 {
          tunnel: w2377 -> [_ w2400]
          frame False {
          }
          frame True {
            n653 = local read "Labstep API_Key"() -> (w2401:string)
            n654 = local read "User"() -> (w2399:string)
            n655 = Concatenate Strings(w2399, " made a logbook entry" ("string")) -> (w2397:string)
            n656 = call "postToLabstepTimeline.vi"("API Key"=w2401, "Post contents"=w2400, "Post title"=w2397) -> ("error out"=w2396:errorcluster)  [unwired: 8 in]
            n657 = Unbundle By Name(w2396) -> ("status"=w2395:bool)
            n658 = case shown="True" w2395 {
              frame False {
                n659 = One Button Dialog(message="Posted! ") -> ()  [unwired: 1 in, 1 out]
              }
              frame True {
                n660 = One Button Dialog(message="Sorry, there was an error posting to the logbook.\nPlease check your connection and try again... ") -> ()  [unwired: 1 in, 1 out]
              }
            }
          }
        }
        n661 = local write "Post to logbook"(FALSE ("Post to logbook")) -> ()
      }
      event "ASI Set Lock": Value Change {
        n662 = event-data() -> ("NewVal"=w2409:bool)  [unwired: 1 in, 5 out]
        n663 = case shown="False" w2409 {
          tunnel: w2408 -> [w2424 w2426]
          tunnel: [w2424 w2429] -> w2407
          tunnel: w2406 -> [w2425 w2427]
          tunnel: [w2425 w2428] -> w2405
          frame False {
          }
          frame True {
            n664 = call "Lock focus.vi"("error in"=w2426, "VISA resource in"=w2427) -> ("error out"=w2429:errorcluster, "VISA resource out"=w2428:refnum<visa-resource-name>)  [unwired: 8 in]
          }
        }
        n665 = local write "ASI Set Lock"(FALSE) -> ()
      }
      event "ASI Unlock": Value Change {
        n666 = event-data() -> ("NewVal"=w2435:bool)  [unwired: 1 in, 5 out]
        n667 = case shown="False" w2435 {
          tunnel: w2432 -> [w2451 w2452]
          tunnel: w2434 -> [w2450 w2453]
          tunnel: [w2451 w2455] -> w2431
          tunnel: [w2450 w2454] -> w2433
          frame False {
          }
          frame True {
            n668 = call "Unlock focus.vi"("error in"=w2453, "VISA resource in"=w2452) -> ("error out"=w2454:errorcluster, "VISA resource out"=w2455:refnum<visa-resource-name>)  [unwired: 8 in]
          }
        }
        n669 = local write "ASI Unlock"(FALSE ("ASI Unlock")) -> ()
      }
      event "LED intensity": Value Change {
        n670 = event-data() -> ("NewVal"=w2457:dbl)  [unwired: 1 in, 5 out]
        n671 = call "Set ASI LED power.vi"("error in"=w2459, "New LED power"=w2457, "VISA resource in"=w2461) -> ("error out"=w2458:errorcluster, "VISA resource name out"=w2460:refnum<visa-resource-name>)  [unwired: 7 in]
      }
      event "TIRF Info button": Value Change {
        n672 = event-data() -> ("NewVal"=w2477:bool)  [unwired: 1 in, 5 out]
        n673 = case shown="True" w2477 {
          frame False {
          }
          frame True {
            n674 = One Button Dialog(message="For the 100X lens, ticking the checkbox will enable TIRF for 488 and 640\nimaging. For the 60X objective, ticking the checkbox should give you\nincreased resolution for 488 and 640, although reconstructions may\nbe noisier - so it's only recommended for well labelled samples. ") -> ()  [unwired: 1 in, 1 out]
          }
        }
        n675 = local write "TIRF Info button"(FALSE ("TIRF Info button")) -> ()
      }
    }
    n676 = Or(x=w159, y="stop") -> (x .or. y?=w161:bool)
  }
  n677 = flat-sequence {
    tunnel: w49 -> [w2523]
    tunnel: w47 -> [w2522]
    tunnel: w45 -> [w2521]
    tunnel: w44 -> [w2520]
    tunnel: w41 -> [w2519]
    tunnel: w40 -> [w2518]
    tunnel: w38 -> [w2517]
    tunnel: w37 -> [w2515]
    tunnel: w27 -> [w2499]
    tunnel: w26 -> [w2514]
    tunnel: w23 -> [w2511]
    tunnel: w22 -> [w2510]
    tunnel: w21 -> [w2506]
    tunnel: w20 -> [_]
    tunnel: [w2503] -> _
    tunnel: w18 -> [w2503]
    tunnel: [w2498] -> w6
    tunnel: w1 -> [w2495]
    tunnel: [w2495] -> w5
    tunnel: w3 -> [w2494]
    tunnel: [w2494] -> w2
    tunnel: w6 -> [w2535]
    tunnel: w5 -> [w2528]
    tunnel: w2 -> [w2524]
    frame #0 {
      w2496 = bool[] [FALSE, FALSE, FALSE] ("data")
      # "ASI VISA"
      # "Bye bye ASI..."
      # "z-pos DAC set"
      # "ASI errors (clustered)"
      # "SLM USB"
      # "SLM trigger"
      # "Camera trig. ready"
      # "Camera ext trig out"
      # "Pockels cell"
      # "Filter wheell (VISA)"
      # "Final tasks"
      # "Turn off all lasers"
      # "Gather and display errors"
      n678 = call "ASI_Disable_Enable_Controls.vi"("Enable Z"=TRUE ("Disable Z"), "error in"=w2499, "Enable XY"=TRUE ("Disable Z"), "VISA resource name"=w2503) -> ("error out"=w2501:errorcluster, "VISA resource name out"=w2502:refnum<visa-resource-name>)
      n679 = Array To Cluster(array=w2496) -> (cluster=w2497:T12)
      n680 = call <vilib>:"DAQmx Clear Task.vi"("task in"=w2523, "error in"=w2522) -> ("error out"=w2507:errorcluster)  [unwired: 13 in]
      n681 = call <vilib>:"DAQmx Clear Task.vi"("task in"=w2520, "error in"=w2521) -> ("error out"=w2508:errorcluster)  [unwired: 13 in]
      n682 = call <vilib>:"DAQmx Clear Task.vi"("task in"=w2517, "error in"=w2515) -> ("error out"=w2516:errorcluster)  [unwired: 13 in]
      n683 = call <vilib>:"DAQmx Clear Task.vi"("task in"=w2519, "error in"=w2518) -> ("error out"=w2505:errorcluster)  [unwired: 13 in]
      n684 = VISA Close(VISA resource name=w2502, error in (no error)=w2501) -> (error out=w2500:errorcluster)
      n685 = call-poly <vilib>:"DAQmx Write.vi"("task/channels in"=w2511, "data"=w2496, "error in"=w2510) -> ("error out"=w2509:errorcluster)  [unwired: 10 in, 2 out]
      n686 = local write "Laser Cluster"(w2497) -> ()
      n687 = call <userlib>:"close Device.vi"("error in (no error)"=w2514) -> ("error out"=w2504:errorcluster)  [unwired: 9 in, 1 out]
      n688 = Merge Errors(w2507, w2508, w2516, w2509, w2506, w2505, w2500, w2504) -> (w2498:errorcluster)
      n689 = call <vilib>:"Simple Error Handler.vi"("error in (no error)"=w2498) -> ()  [unwired: 4 in, 5 out]
    }
    frame #1 {
      w2536 = FALSE
      # "Log any errors to the Labstep log book"
      # "Post to Labstep"
      # "Flick stop switch back off for next run"
      n690 = Unbundle By Name(w2535) -> ("source"=w2529:string, "status"=w2530:bool)
      n691 = local write "stop"(w2536) -> ()
      n692 = local write "Acquire"(w2536) -> ()
      n693 = local write "Live on"(w2536) -> ()
      n694 = local read "Labstep API_Key"() -> (w2526:string)
      n695 = Concatenate Strings("The error handler reported the following error: " ("string"), "\n", w2529) -> (w2531:string)
      n696 = Select(t=w2531, s=w2530, f="The software exited without reporting any errors. " ("string")) -> (s? t:f=w2527:string)
      n697 = call "Add post to experiment.vi"("API Key"=w2526, "Thread ID"=w2524, "Post contents"=w2527) -> ("error out"=w2525:errorcluster)  [unwired: 8 in]
      n698 = call "End experiment.vi"("API Key"=w2526, "error in"=w2525, "Experiment ID"=w2528) -> ()  [unwired: 8 in, 1 out]
    }
    frame #2 {
      # "Close the window"
      n699 = vi-ref "SIM control.vi"() -> (w2540:refnum<vi>)
      n700 = property class="VI"(reference=w2540) -> ("Name"=w2537:string)  [unwired: 1 in, 2 out]
      n701 = Open VI Reference(vi path=w2537) -> (vi reference=w2539:refnum<vi>)  [unwired: 5 in, 1 out]
      n702 = invoke class="VI" method="FP.Close"(reference=w2539) -> (reference out=w2538:refnum<vi>)  [unwired: 2 in, 2 out]
      n703 = Close Reference(reference=w2538) -> ()  [unwired: 1 in, 1 out]
    }
  }
